vi "SISE-Monitor110-Demo.vi"() -> ()   [LabVIEW 2024]
uses:
  Labview-Projects2019/IonFluxProgramms2019/IonFluxMonitor/SubVIs-SISE-Monitor/Control-IonFlux.ctl
  <vilib>/DAQmx/create/channels.llb/DAQmx Create Channel (AI-Voltage-Basic).vi
  <vilib>/Instr/_visa.llb/VISA Configure Serial Port (Instr).vi
  <vilib>/Analysis/NI_AALPro.lvlib
  <vilib>/DAQmx/read.llb/DAQmx Read (Analog 2D DBL NChan NSamp).vi
panel:
  out "Lesepuffer":string
  out "Registerkarte":enum32{"Start", "Record", "Stop"}(tab)
  out "Output V ch 2":bool
  in  "V channel 2":bool
  out "Output V ch 1":bool
  in  "V channel 1":bool
  out "SISE channel 1":bool
  out "Output SISE ch 2":bool
  in  "SISE channel 2":bool
  out "slow":bool
  in  "Scan angle (degrees)":dbl(slide) scale=0.0..90.0
  out "?":dbl
  in  "VISA res. name":refnum<visa-resource-name> caption="VISA-Ressourcenname"
  in  "Start measurement":bool
  out "Data File":bool
  out "Ind. Channel In":bool
  in  "Data file":path
  out "Ind. Channel Out":bool
  out "?":dbl
  out "Record period (round at 5s)":dbl
  in  "Scan distance (µm)":dbl(slide)=50.0 scale=0.0..100.0
  in  "Record period (single track, s)":dbl(slide)=10.112359550561797 scale=0.0..60.0 scale format="%#_2f"
  in  "Manipulator Speed":bool
  out "fast":bool
  in  "Channels In":tag
  in  "Position of manipulator":bool
  out "left":bool
  out "right":bool
  in  "TC 3":T1(tab)
  in  "Range limit\nS1.1 (mV)":dbl(slide)=200.0 min=0.0 max=600.0 scale=0.2..600.0
  in  "Base line\nS1.1 (mV)":dbl(slide) scale=-300.0..300.0
  in  "Range limit\nS1.2 mV":dbl(slide)=30.0 scale=0.1..30.0
  in  "Base line \nS1.2 (mV)":dbl(slide) scale=-15.0..15.0
  out "dV-SISE channel 1":cluster{dbl[], dbl[]}[](graph)
  out "V-SISE channel 1":cluster{dbl[], dbl[]}[](graph)
  out "V-SISE channel 2":cluster{dbl[], dbl[]}[](graph)
  out "dV-SISE channel 2":cluster{dbl[], dbl[]}[](graph)
  in  "Range limit\nS2.1 (mV)":dbl(slide)=200.0 min=0.0 max=600.0 scale=0.2..600.0
  in  "Base line\nS2.1 (mV)":dbl(slide) scale=-300.0..300.0
  in  "Base line \nS2.2 (mV)":dbl(slide) scale=-15.0..15.0
  in  "Range limit\nS2.2 (mV)":dbl(slide)=30.0 scale=0.1..30.0
  out "Voltage channel 1":cluster{dbl[], dbl[]}[](graph)
  in  "Base line\nV1 (V)":dbl(slide) scale=-300.0..300.0
  in  "Range limit\nV1 (V)":dbl(slide)=200.0 min=0.0 max=600.0 scale=0.2..600.0
  in  "Base line\nV2 (V)":dbl(slide) scale=-300.0..300.0
  in  "Range limit\nV2 (V)":dbl(slide)=200.0 min=0.0 max=600.0 scale=0.2..600.0
  out "Voltage channel 2":cluster{dbl[], dbl[]}[](graph)
  out "V channel #2":bool
  out "V channel #1":bool
  out "SISE channel #2":bool
  out "SISE channel #1":bool
  in  "?":T2(tab)
  in  "V SISE\nch #1":dbl(slide)=4.96774193548387 scale=-10.0..10.0
  out "Vprobe SISE 1":cluster{dbl[], dbl[]}[](graph)
  in  "V SISE\nch #2":dbl(slide)=4.96774193548387 scale=-10.0..10.0
  out "Vprobe SISE 2":cluster{dbl[], dbl[]}[](graph)
  in  "Vch #1":dbl(slide)=5.096774193548386 scale=-10.0..10.0
  out "Vprobe V 1":cluster{dbl[], dbl[]}[](graph)
  in  "Vch\n#2":dbl(slide)=5.096774193548386 scale=-10.0..10.0
  out "Vprobe V 2":cluster{dbl[], dbl[]}[](graph)
  in  "Enable change position 0":bool
  out "Raw data file":path
  in  "Stop measurent":bool
  out "Position probe":cluster{dbl[], dbl[]}[](graph)
  in  "Add Mark":bool
  in  "Event Mark":string
  out "Stop recording":bool
  out "String":string
  out "E-mark on":T3
  out "?":string
  in  "Bildlaufleiste":i32(c297)
  in  "Start fit (% of rec. period)":dbl(slide)=50.0 scale=0.0..100.0
  in  "?":enum32{"dV SISE 1", "dV SISE 2"}(tab)
  out "deltaV SISE 1":cluster{dbl[], "Best Linear Fit":dbl[]}[](graph)
  out "deltaV SISE 2":cluster{dbl[], "Best Linear Fit":dbl[]}[](graph)
  in  "Zoom from start":dbl(slide) scale=0.0..100.0
  in  "Zoom from end":dbl(slide)=100.0 scale=0.0..100.0
  in  "Stop programm":bool
  in  "New measurement":bool
  out "Stop recording 2":bool
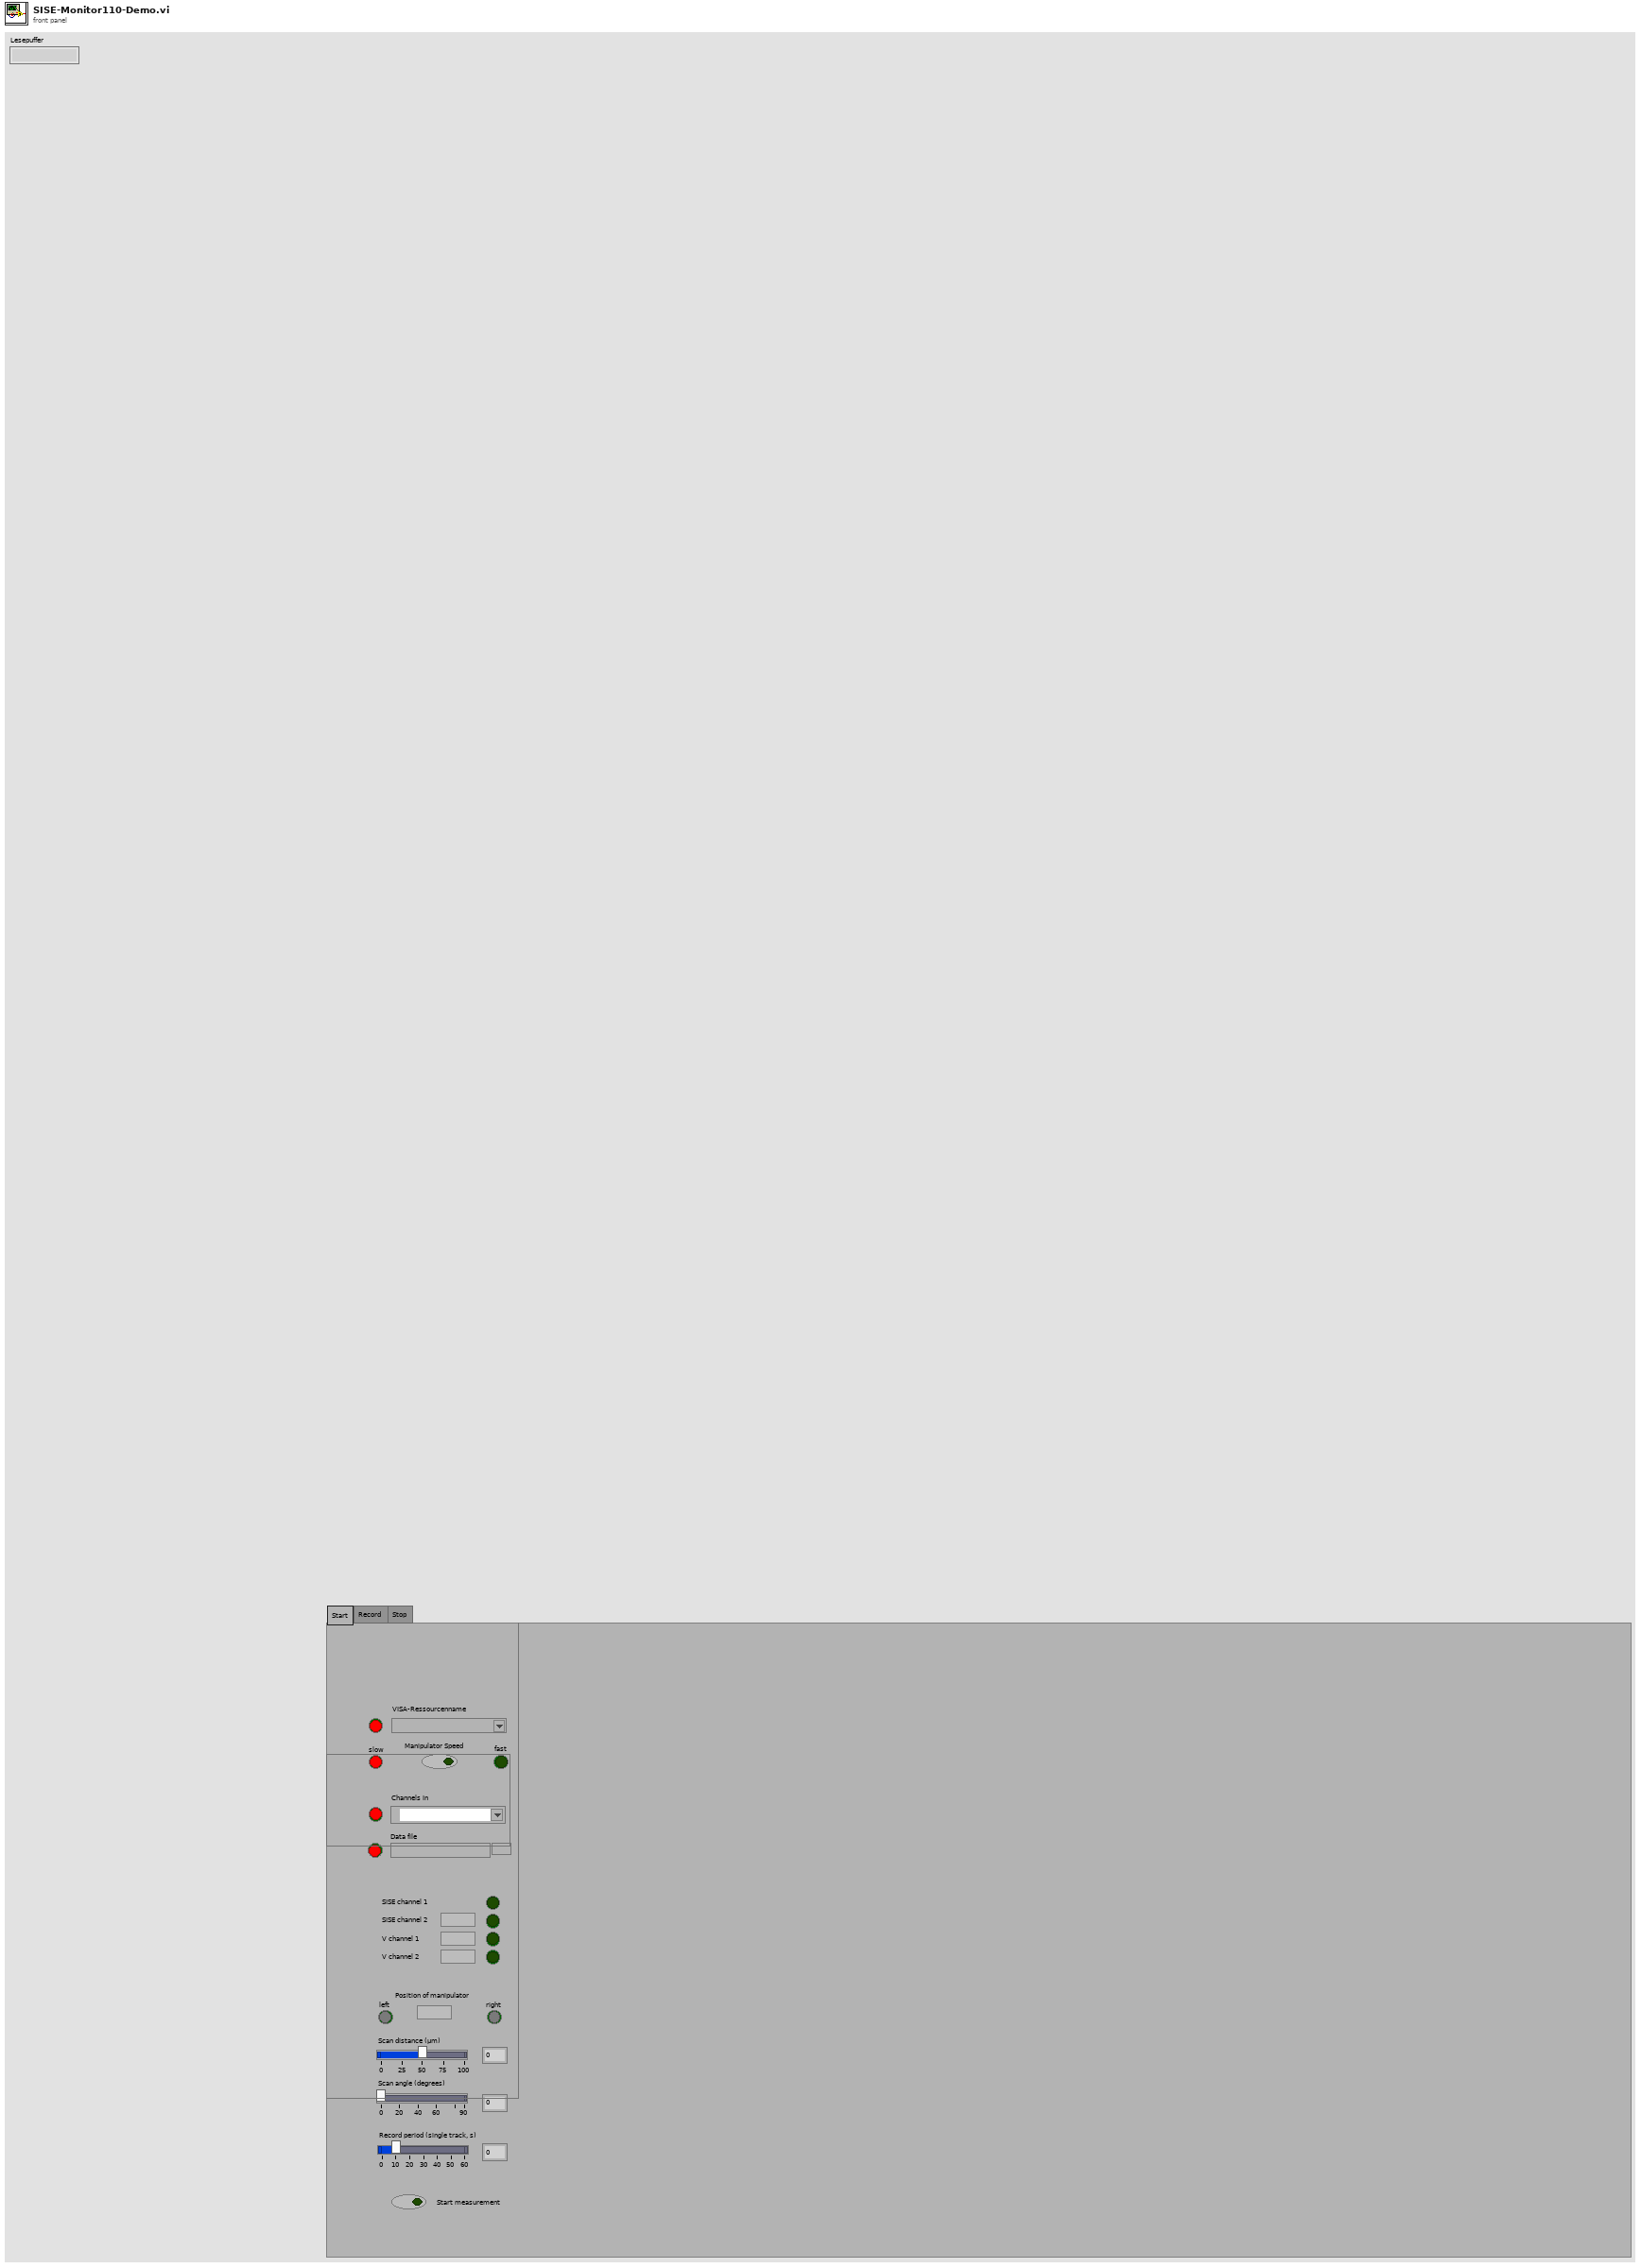
[diagram p1: front panel]
types:
  T1 = enum32{"SISE channel #1", "SISE channel #2", "V channel #1", "V channel #2"}
  T2 = enum32{"SISE chan #1", "SISE chan #2", "V chan #1", "V chan #2"}
  T3 = typedef "Control-IonFlux.ctl" = bool
  T4 = cluster{"refnum out":refnum<file>, "status":bool, "code":i32, "source":string}
  T5 = cluster{"task out":refnum<k21>, "status":bool, "code":i32, "source":string}
  T6 = enum16{"open", "replace", "create", "open or create", "replace or create", "replace or create with confirmation"}
  T7 = cluster{"refnum":refnum<file>, "status":bool, "code":i32, "source":string}
  T8 = cluster{dbl[], dbl[], "Best Linear Fit":dbl[], dbl[], dbl[]}
  T9 = cluster{"Array (Ausgang)":dbl[], "Array (Ausgang)":dbl[]}
  T10 = cluster{"Array (Ausgang)":dbl[], "Array (Ausgang)":dbl[]}[]
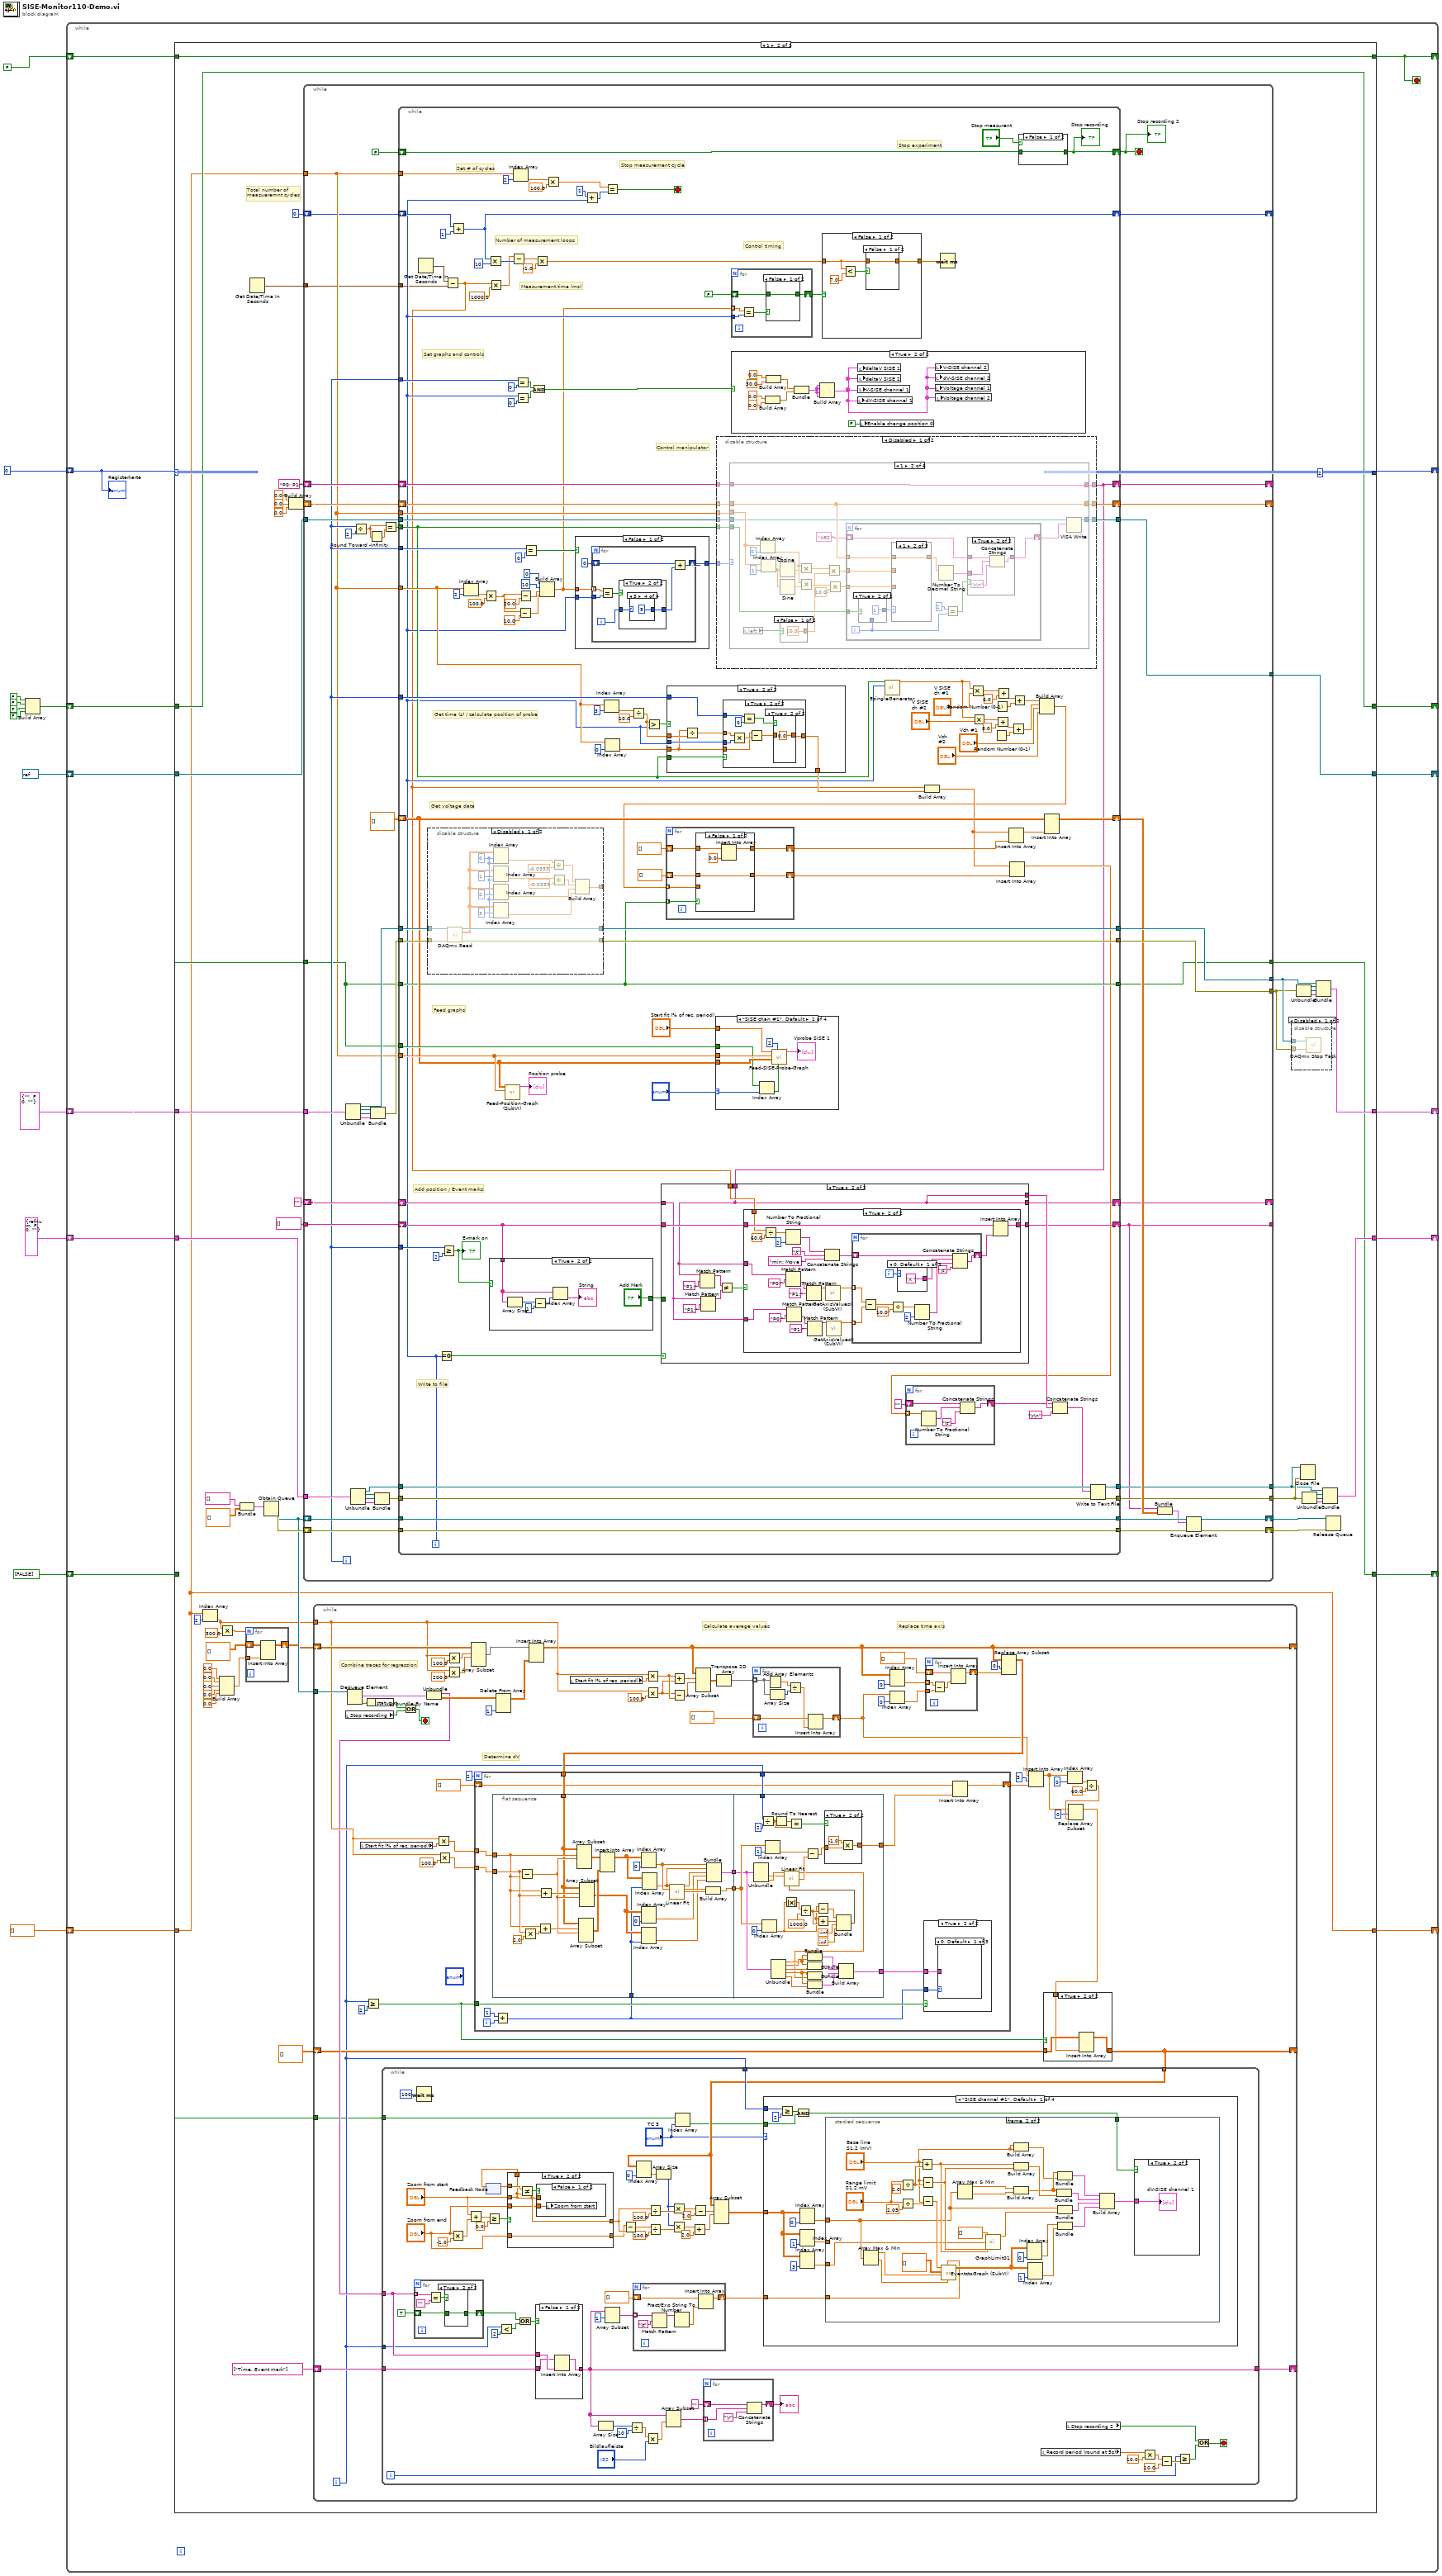
[diagram p0: block diagram]
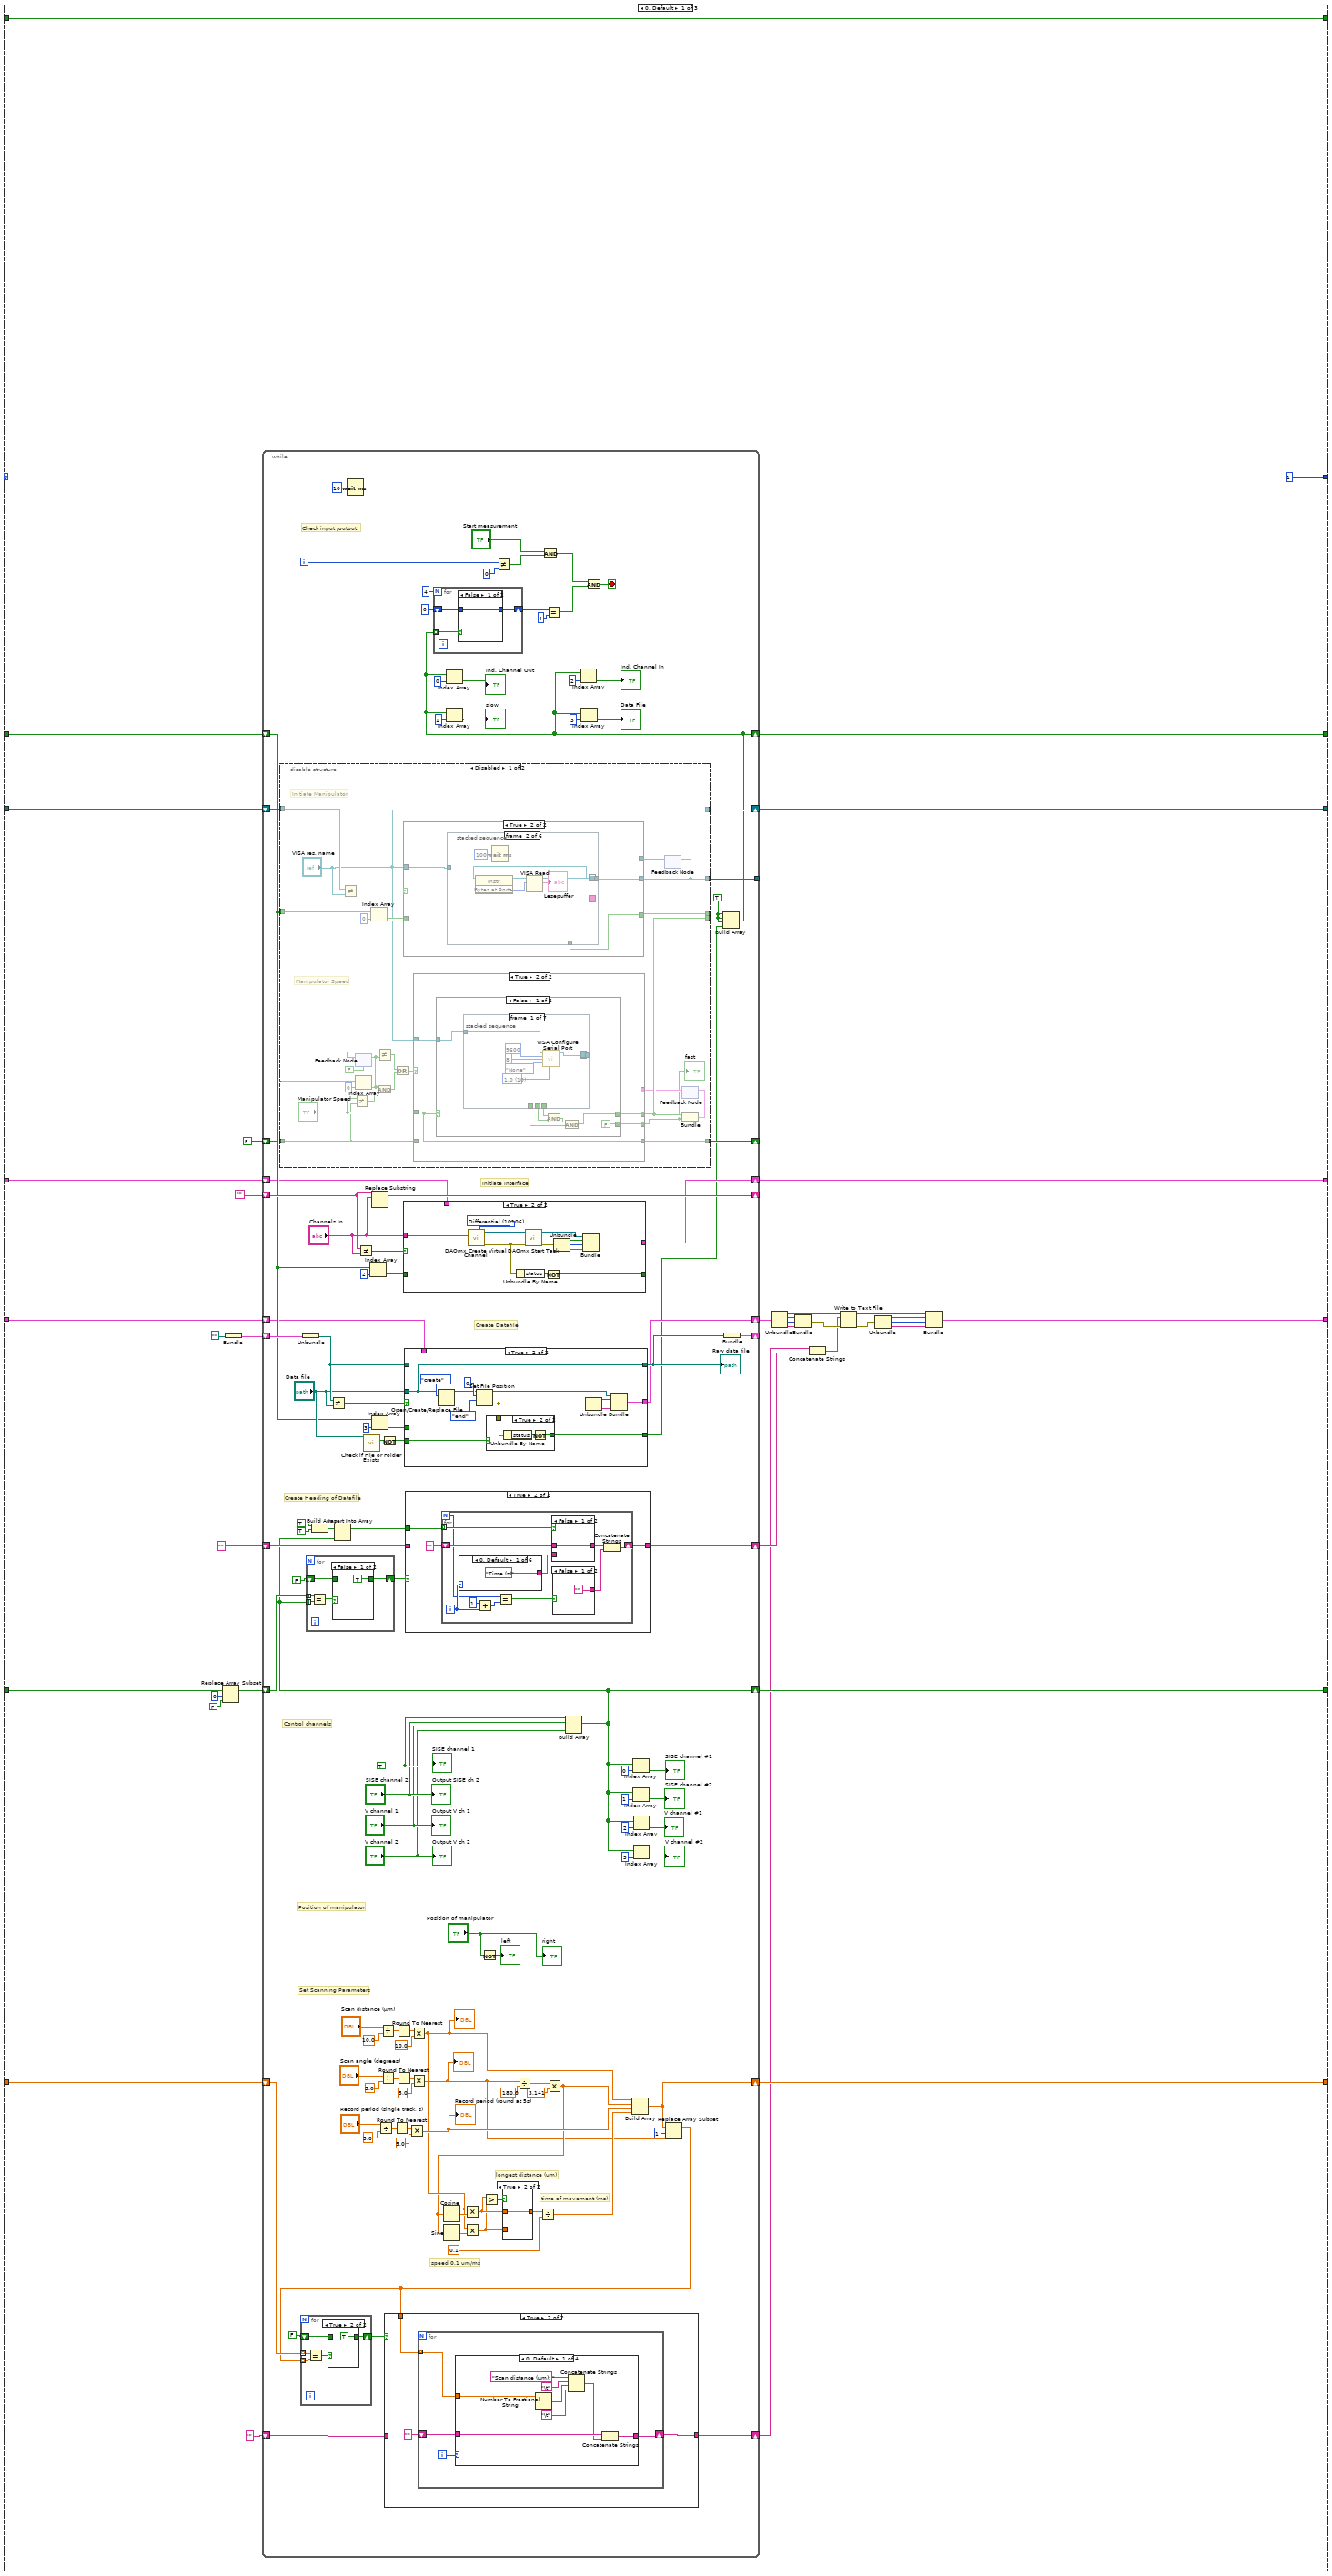
[diagram p2: hidden frame]
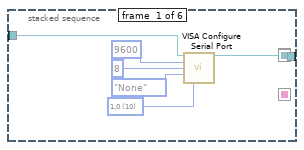
[diagram p4: hidden frame]
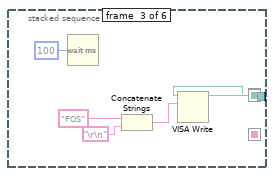
[diagram p5: hidden frame]
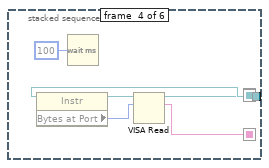
[diagram p6: hidden frame]
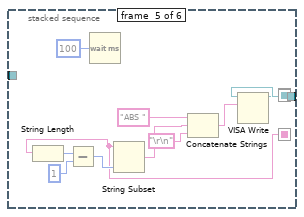
[diagram p7: hidden frame]
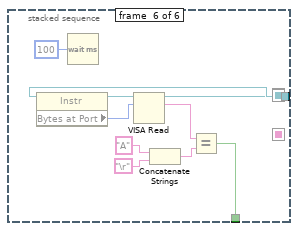
[diagram p8: hidden frame]
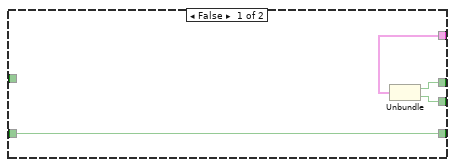
[diagram p9: hidden frame]
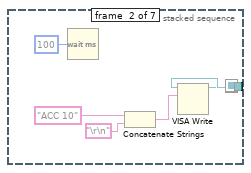
[diagram p10: hidden frame]
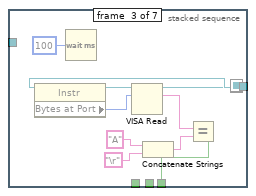
[diagram p11: hidden frame]
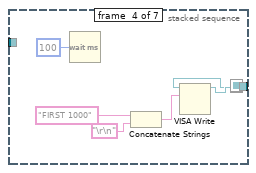
[diagram p12: hidden frame]
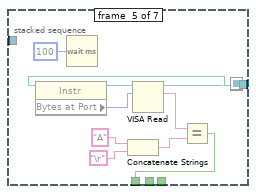
[diagram p13: hidden frame]
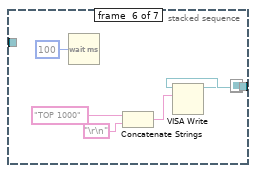
[diagram p14: hidden frame]
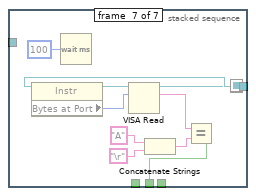
[diagram p15: hidden frame]
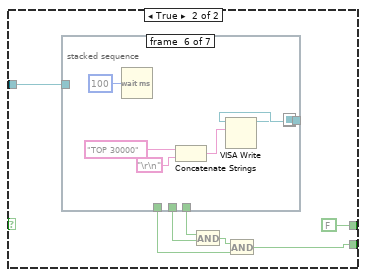
[diagram p16: hidden frame]
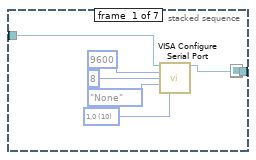
[diagram p17: hidden frame]
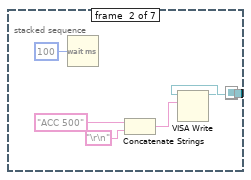
[diagram p18: hidden frame]
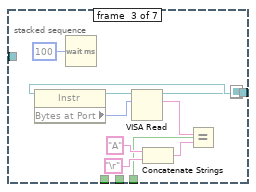
[diagram p19: hidden frame]
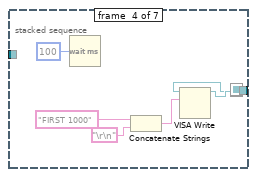
[diagram p20: hidden frame]
diagram:
  n1 = Build Array(FALSE, FALSE, FALSE, FALSE) -> (w1:bool[])
  n2 = while {
    shift-right: [w28] -> _
    shift-left: 0 -> [w27]
    shift-right: [w25] -> _
    shift-left: refnum<visa-resource-name> refnum ("VISA res. name") -> [w26]
    shift-right: [w23] -> _
    shift-left: T5 {"task out"="", "status"=FALSE, "code"=0, "source"=""} -> [w24]
    shift-right: [w19] -> _
    shift-left: T4 {"refnum out"=refnum, "status"=FALSE, "code"=0, "source"=""} -> [w20]
    shift-right: [w22] -> _
    shift-left: dbl[] [] -> [w21]
    shift-right: [w18] -> _
    shift-left: bool[] [FALSE] -> [w17]
    shift-right: [w15] -> _
    shift-left: FALSE -> [w16]
    shift-right: [w13] -> _
    shift-left: w1 -> [w14]
    stop <- w15 stop-if-true
    n3 = case shown="1" w27 {
      tunnel: [1 2 0] -> w28
      tunnel: w26 -> [w60 w561 w1653]
      tunnel: [w59 w560 w1653] -> w25
      tunnel: w24 -> [w58 w559 w1652]
      tunnel: [w57 w555 w1652] -> w23
      tunnel: [w40 w535 w1650] -> w19
      tunnel: w20 -> [w56 w539 w1650]
      tunnel: [w55 w518 w1651] -> w22
      tunnel: w21 -> [w54 w518 w1651]
      tunnel: w17 -> [w31 w525 w1649]
      tunnel: [w53 w532 w1649] -> w18
      tunnel: w16 -> [w39 w524 w1648]
      tunnel: [w39 w524 w1647] -> w15
      tunnel: w14 -> [w33 w523 w1646]
      tunnel: [w38 w523 w1646] -> w13
      frame 0, Default {
        n4 = Replace Array Subset(array=w31, new element=FALSE ("Neues Element/Teil-Array"), index=0 ("Index")) -> (w32:bool[])
        n5 = Bundle(path "") -> (w61:cluster{path})  [unwired: 1 in]
        n6 = while {
          shift-right: [w117] -> w59
          shift-left: w60 -> [w165]
          shift-right: [w90] -> w38
          shift-left: w33 -> [w123]
          tunnel: [w124] -> _
          shift-right: [w160] -> _
          shift-left: "" -> [w159]
          shift-right: [w151] -> _
          shift-left: w61 -> [w153]
          shift-right: [w118] -> _
          shift-left: FALSE -> [w122]
          shift-right: [w115] -> w57
          shift-left: w58 -> [w116]
          shift-right: [w113] -> w51
          shift-left: w56 -> [w112]
          shift-right: [w73] -> w55
          shift-left: w54 -> [w77]
          shift-right: [w82] -> w53
          shift-left: w32 -> [w85]
          shift-right: [w87] -> w36
          shift-left: "" -> [w86]
          shift-right: [w79] -> w35
          shift-left: "" -> [w75]
          i -> [w80]
          stop <- w83 stop-if-true
          w68 = TRUE
          w108 = TRUE
          # "Position of manipulator"
          # "Set Scanning Parameters"
          # "Control channels"
          # "Create Heading of Datafile"
          # "Create Datafile"
          # "Initiate Interface"
          # "Check input /output"
          # "speed 0.1 um/ms"
          # "longest distance (um)"
          # "time of movement (ms)"
          n7 = disable-structure shown="Disabled" {
            disable-tunnel: w165 -> [w200 _]
            disable-tunnel: [w196 _] -> w124
            disable-tunnel: w123 -> [w194 _]
            disable-tunnel: w122 -> [w191 _]
            disable-tunnel: [w184 _] -> _
            disable-tunnel: [w183 _] -> _
            disable-tunnel: [w180 _] -> w118
            disable-tunnel: ["VISA res. name" _] -> w117
            frame Disabled {
              # "Manipulator Speed"
              # "Initiate Manipulator"
              n8 = Not Equal?(x=w200, y="VISA res. name") -> (x != y?=w177:bool)
              n9 = Not Equal?(x="Manipulator Speed", y=w191) -> (x != y?=w193:bool)
              n10 = feedback #1(FALSE) -> (w188:bool)
              n11 = Index Array(array=w194, index=0 ("Index")) -> (element=w189:bool)
              n12 = feedback-in #1(w189) -> ()
              n13 = Index Array(array=w194, index=0 ("Index")) -> (element=w198:bool)
              n14 = Not Equal?(x=w188, y=w189) -> (x != y?=w187:bool)
              n15 = And(x=w189, y=w193) -> (x .and. y?=w185:bool)
              n16 = Or(x=w187, y=w185) -> (x .or. y?=w186:bool)
              n17 = feedback #2() -> (w197:refnum<visa-resource-name>)  [unwired: 1 in]
              n18 = case shown="True" w177 {
                tunnel: w198 -> [w202 _]
                tunnel: [w202 w205] -> w184
                tunnel: "VISA res. name" -> [_ w204]
                tunnel: [w201 w203] -> w196
                tunnel: w197 -> [w201 _]
                frame False {
                }
                frame True {
                  n19 = stacked-sequence {
                    seq-local: [w206 _ _ _ _ _] -> [_ w213 _ _ _ _]
                    seq-local: [_ w214 _ _ _ _] -> [_ _ w218 _ _ _]
                    seq-local: [_ _ w219 _ _ _] -> [_ _ _ w226 _ _]
                    seq-local: [_ _ _ w225 _ _] -> [_ _ _ _ w237 _]
                    seq-local: [_ _ _ w224 _ _] -> [_ _ _ _ w231 _]
                    seq-local: [_ _ _ _ w236 _] -> [_ _ _ _ _ w247]
                    tunnel: w204 -> [w211 _ _ _ _ _]
                    tunnel: [_ _ _ _ _ w246] -> w203
                    tunnel: [_ _ _ _ _ w241] -> w205
                    frame #0 {
                      w207 = u16 10 items=["1,0"=10, "1,5"=15, "2,0"=20] ("stop bits (10: 1 bit)")
                      n20 = call-poly "VISA Configure Serial Port"("VISA resource name"=w211, "baud rate (9600)"=u32 9600, "data bits (8)"=u16 8, "parity (0:none)"=enum16{"None", "Odd", "Even", "Mark", "Space"}."None", "stop bits (10: 1 bit)"=w207) -> ("VISA resource name out"=w206:refnum<visa-resource-name>)  [unwired: 9 in, 1 out]
                    }
                    frame #1 {
                      n21 = property class="Instr"(reference=w213) -> (reference out=w216:refnum<visa-resource-name>, "Bytes at Port"=w215:u32)  [unwired: 1 in, 1 out]
                      n22 = Wait (ms)(milliseconds to wait=u32 100) -> ()  [unwired: 1 out]
                      n23 = VISA Read(VISA resource name=w216, byte count=w215) -> (VISA resource name out=w214:refnum<visa-resource-name>, read buffer=→"Lesepuffer":string)  [unwired: 1 in, 2 out]
                    }
                    frame #2 {
                      n24 = Wait (ms)(milliseconds to wait=u32 100) -> ()  [unwired: 1 out]
                      n25 = Concatenate Strings("POS", "\r\n") -> (w220:string)
                      n26 = VISA Write(VISA resource name=w218, write buffer=w220) -> (VISA resource name out=w219:refnum<visa-resource-name>)  [unwired: 1 in, 2 out]
                    }
                    frame #3 {
                      n27 = property class="Instr"(reference=w226) -> (reference out=w227:refnum<visa-resource-name>, "Bytes at Port"=w228:u32)  [unwired: 1 in, 1 out]
                      n28 = Wait (ms)(milliseconds to wait=u32 100) -> ()  [unwired: 1 out]
                      n29 = VISA Read(VISA resource name=w227, byte count=w228) -> (VISA resource name out=w225:refnum<visa-resource-name>, read buffer=w224:string)  [unwired: 1 in, 2 out]
                    }
                    frame #4 {
                      n30 = String Length(string=w231) -> (length=w234:i32)
                      n31 = Subtract(x=w234, y=1) -> (x-y=w232:i32)
                      n32 = Wait (ms)(milliseconds to wait=u32 100) -> ()  [unwired: 1 out]
                      n33 = String Subset(string=w231, length (rest)=w232) -> (substring=w230:string)  [unwired: 1 in]
                      n34 = Concatenate Strings("ABS ", w230, "\r\n") -> (w238:string)
                      n35 = VISA Write(VISA resource name=w237, write buffer=w238) -> (VISA resource name out=w236:refnum<visa-resource-name>)  [unwired: 1 in, 2 out]
                    }
                    frame #5 {
                      n36 = property class="Instr"(reference=w247) -> (reference out=w248:refnum<visa-resource-name>, "Bytes at Port"=w249:u32)  [unwired: 1 in, 1 out]
                      n37 = Wait (ms)(milliseconds to wait=u32 100) -> ()  [unwired: 1 out]
                      n38 = VISA Read(VISA resource name=w248, byte count=w249) -> (VISA resource name out=w246:refnum<visa-resource-name>, read buffer=w242:string)  [unwired: 1 in, 2 out]
                      n39 = Concatenate Strings("A", "\r") -> (w245:string)
                      n40 = Equal?(x=w242, y=w245) -> (x = y?=w241:bool)
                    }
                  }
                }
              }
              n41 = feedback-in #2(w196) -> ()
              n42 = feedback #3() -> (w181:cluster{bool, bool})  [unwired: 1 in]
              n43 = case shown="True" w186 {
                tunnel: "VISA res. name" -> [_ w258]
                tunnel: [w254 w257] -> w180
                tunnel: "Manipulator Speed" -> [_ w257]
                tunnel: w191 -> [w254 _]
                tunnel: [w251 w256] -> w183
                tunnel: [w252 w255] -> w178
                tunnel: w181 -> [w253 _]
                frame False {
                  n44 = Unbundle(w253) -> (w251:bool, w252:bool)
                }
                frame True {
                  n45 = case shown="False" w257 {
                    tunnel: w258 -> [w265 w326]
                    tunnel: [FALSE w320] -> w255
                    tunnel: [w259 FALSE] -> w256
                    frame False {
                      n46 = stacked-sequence {
                        seq-local: [w266 _ _ _ _ _ _] -> [_ w276 _ _ _ _ _]
                        seq-local: [_ w272 _ _ _ _ _] -> [_ _ w285 _ _ _ _]
                        seq-local: [_ _ w279 _ _ _ _] -> [_ _ _ w288 _ _ _]
                        seq-local: [_ _ _ w289 _ _ _] -> [_ _ _ _ w300 _ _]
                        seq-local: [_ _ _ _ w299 _ _] -> [_ _ _ _ _ w305 _]
                        seq-local: [_ _ _ _ _ w304 _] -> [_ _ _ _ _ _ w316]
                        tunnel: w265 -> [w271 _ _ _ _ _ _]
                        tunnel: [_ _ w278 _ _ _ _] -> w263
                        tunnel: [_ _ _ _ w294 _ _] -> w261
                        tunnel: [_ _ _ _ _ _ w315] -> _
                        tunnel: [_ _ _ _ _ _ w310] -> w262
                        frame #0 {
                          w267 = u16 10 items=["1,0"=10, "1,5"=15, "2,0"=20] ("stop bits (10: 1 bit)")
                          n47 = call-poly "VISA Configure Serial Port"("VISA resource name"=w271, "baud rate (9600)"=u32 9600, "data bits (8)"=u16 8, "parity (0:none)"=enum16{"None", "Odd", "Even", "Mark", "Space"}."None", "stop bits (10: 1 bit)"=w267) -> ("VISA resource name out"=w266:refnum<visa-resource-name>)  [unwired: 9 in, 1 out]
                        }
                        frame #1 {
                          n48 = Wait (ms)(milliseconds to wait=u32 100) -> ()  [unwired: 1 out]
                          n49 = Concatenate Strings("ACC 10", "\r\n") -> (w273:string)
                          n50 = VISA Write(VISA resource name=w276, write buffer=w273) -> (VISA resource name out=w272:refnum<visa-resource-name>)  [unwired: 1 in, 2 out]
                        }
                        frame #2 {
                          n51 = property class="Instr"(reference=w285) -> (reference out=w286:refnum<visa-resource-name>, "Bytes at Port"=w284:u32)  [unwired: 1 in, 1 out]
                          n52 = Wait (ms)(milliseconds to wait=u32 100) -> ()  [unwired: 1 out]
                          n53 = VISA Read(VISA resource name=w286, byte count=w284) -> (VISA resource name out=w279:refnum<visa-resource-name>, read buffer=w283:string)  [unwired: 1 in, 2 out]
                          n54 = Concatenate Strings("A", "\r") -> (w280:string)
                          n55 = Equal?(x=w283, y=w280) -> (x = y?=w278:bool)
                        }
                        frame #3 {
                          n56 = Wait (ms)(milliseconds to wait=u32 100) -> ()  [unwired: 1 out]
                          n57 = Concatenate Strings("FIRST 1000", "\r\n") -> (w290:string)
                          n58 = VISA Write(VISA resource name=w288, write buffer=w290) -> (VISA resource name out=w289:refnum<visa-resource-name>)  [unwired: 1 in, 2 out]
                        }
                        frame #4 {
                          n59 = property class="Instr"(reference=w300) -> (reference out=w301:refnum<visa-resource-name>, "Bytes at Port"=w302:u32)  [unwired: 1 in, 1 out]
                          n60 = Wait (ms)(milliseconds to wait=u32 100) -> ()  [unwired: 1 out]
                          n61 = Concatenate Strings("A", "\r") -> (w295:string)
                          n62 = VISA Read(VISA resource name=w301, byte count=w302) -> (VISA resource name out=w299:refnum<visa-resource-name>, read buffer=w298:string)  [unwired: 1 in, 2 out]
                          n63 = Equal?(x=w298, y=w295) -> (x = y?=w294:bool)
                        }
                        frame #5 {
                          n64 = Wait (ms)(milliseconds to wait=u32 100) -> ()  [unwired: 1 out]
                          n65 = Concatenate Strings("TOP 1000", "\r\n") -> (w306:string)
                          n66 = VISA Write(VISA resource name=w305, write buffer=w306) -> (VISA resource name out=w304:refnum<visa-resource-name>)  [unwired: 1 in, 2 out]
                        }
                        frame #6 {
                          n67 = property class="Instr"(reference=w316) -> (reference out=w317:refnum<visa-resource-name>, "Bytes at Port"=w318:u32)  [unwired: 1 in, 1 out]
                          n68 = Wait (ms)(milliseconds to wait=u32 100) -> ()  [unwired: 1 out]
                          n69 = VISA Read(VISA resource name=w317, byte count=w318) -> (VISA resource name out=w315:refnum<visa-resource-name>, read buffer=w311:string)  [unwired: 1 in, 2 out]
                          n70 = Concatenate Strings("A", "\r") -> (w314:string)
                          n71 = Equal?(x=w311, y=w314) -> (x = y?=w310:bool)
                        }
                      }
                      n72 = And(x=w263, y=w262) -> (x .and. y?=w264:bool)
                      n73 = And(x=w264, y=w261) -> (x .and. y?=w259:bool)
                    }
                    frame True {
                      n74 = stacked-sequence {
                        seq-local: [w327 _ _ _ _ _ _] -> [_ w337 _ _ _ _ _]
                        seq-local: [_ w333 _ _ _ _ _] -> [_ _ w346 _ _ _ _]
                        seq-local: [_ _ w340 _ _ _ _] -> [_ _ _ w349 _ _ _]
                        seq-local: [_ _ _ w350 _ _ _] -> [_ _ _ _ w361 _ _]
                        seq-local: [_ _ _ _ w360 _ _] -> [_ _ _ _ _ w366 _]
                        seq-local: [_ _ _ _ _ w365 _] -> [_ _ _ _ _ _ w377]
                        tunnel: w326 -> [w332 _ _ _ _ _ _]
                        tunnel: [_ _ w339 _ _ _ _] -> w324
                        tunnel: [_ _ _ _ w355 _ _] -> w322
                        tunnel: [_ _ _ _ _ _ w376] -> _
                        tunnel: [_ _ _ _ _ _ w371] -> w323
                        frame #0 {
                          w328 = u16 10 items=["1,0"=10, "1,5"=15, "2,0"=20] ("stop bits (10: 1 bit)")
                          n75 = call-poly "VISA Configure Serial Port"("VISA resource name"=w332, "baud rate (9600)"=u32 9600, "data bits (8)"=u16 8, "parity (0:none)"=enum16{"None", "Odd", "Even", "Mark", "Space"}."None", "stop bits (10: 1 bit)"=w328) -> ("VISA resource name out"=w327:refnum<visa-resource-name>)  [unwired: 9 in, 1 out]
                        }
                        frame #1 {
                          n76 = Wait (ms)(milliseconds to wait=u32 100) -> ()  [unwired: 1 out]
                          n77 = Concatenate Strings("ACC 500", "\r\n") -> (w334:string)
                          n78 = VISA Write(VISA resource name=w337, write buffer=w334) -> (VISA resource name out=w333:refnum<visa-resource-name>)  [unwired: 1 in, 2 out]
                        }
                        frame #2 {
                          n79 = property class="Instr"(reference=w346) -> (reference out=w347:refnum<visa-resource-name>, "Bytes at Port"=w345:u32)  [unwired: 1 in, 1 out]
                          n80 = Wait (ms)(milliseconds to wait=u32 100) -> ()  [unwired: 1 out]
                          n81 = VISA Read(VISA resource name=w347, byte count=w345) -> (VISA resource name out=w340:refnum<visa-resource-name>, read buffer=w344:string)  [unwired: 1 in, 2 out]
                          n82 = Concatenate Strings("A", "\r") -> (w341:string)
                          n83 = Equal?(x=w344, y=w341) -> (x = y?=w339:bool)
                        }
                        frame #3 {
                          n84 = Wait (ms)(milliseconds to wait=u32 100) -> ()  [unwired: 1 out]
                          n85 = Concatenate Strings("FIRST 1000", "\r\n") -> (w351:string)
                          n86 = VISA Write(VISA resource name=w349, write buffer=w351) -> (VISA resource name out=w350:refnum<visa-resource-name>)  [unwired: 1 in, 2 out]
                        }
                        frame #4 {
                          n87 = property class="Instr"(reference=w361) -> (reference out=w362:refnum<visa-resource-name>, "Bytes at Port"=w363:u32)  [unwired: 1 in, 1 out]
                          n88 = Wait (ms)(milliseconds to wait=u32 100) -> ()  [unwired: 1 out]
                          n89 = Concatenate Strings("A", "\r") -> (w356:string)
                          n90 = VISA Read(VISA resource name=w362, byte count=w363) -> (VISA resource name out=w360:refnum<visa-resource-name>, read buffer=w359:string)  [unwired: 1 in, 2 out]
                          n91 = Equal?(x=w359, y=w356) -> (x = y?=w355:bool)
                        }
                        frame #5 {
                          n92 = Wait (ms)(milliseconds to wait=u32 100) -> ()  [unwired: 1 out]
                          n93 = Concatenate Strings("TOP 30000", "\r\n") -> (w367:string)
                          n94 = VISA Write(VISA resource name=w366, write buffer=w367) -> (VISA resource name out=w365:refnum<visa-resource-name>)  [unwired: 1 in, 2 out]
                        }
                        frame #6 {
                          n95 = property class="Instr"(reference=w377) -> (reference out=w378:refnum<visa-resource-name>, "Bytes at Port"=w379:u32)  [unwired: 1 in, 1 out]
                          n96 = Wait (ms)(milliseconds to wait=u32 100) -> ()  [unwired: 1 out]
                          n97 = VISA Read(VISA resource name=w378, byte count=w379) -> (VISA resource name out=w376:refnum<visa-resource-name>, read buffer=w372:string)  [unwired: 1 in, 2 out]
                          n98 = Concatenate Strings("A", "\r") -> (w375:string)
                          n99 = Equal?(x=w372, y=w375) -> (x = y?=w371:bool)
                        }
                      }
                      n100 = And(x=w324, y=w323) -> (x .and. y?=w325:bool)
                      n101 = And(x=w325, y=w322) -> (x .and. y?=w320:bool)
                    }
                  }
                }
              }
              "fast" <- w178
              n102 = Bundle(w183, w178) -> (w182:cluster{bool, bool})  [unwired: 1 in]
              n103 = feedback-in #3(w182) -> ()
            }
            frame Enabled {
            }
          }
          n104 = Unbundle(w153) -> (w152:path)
          n105 = Build Array(TRUE, TRUE) -> (w93:bool[])
          n106 = Not Equal?(x=w152, y="Data file") -> (x != y?=w92:bool)
          n107 = Wait (ms)(milliseconds to wait=u32 10) -> ()  [unwired: 1 out]
          n108 = Not Equal?(x=w159, y="Channels In") -> (x != y?=w162:bool)
          n109 = call <vilib>:"Check if File or Folder Exists.vi"("path"="Data file") -> ("file or folder exists?"=w157:bool)  [unwired: 8 in, 2 out]
          n110 = Index Array(array=w123, index=2 ("Index")) -> (element=w161:bool)
          n111 = Replace Substring(4:"Channels In", 5:w159) -> (1:w160:string)  [unwired: 2 in, 1 out]
          n112 = Index Array(array=w123, index=3 ("Index")) -> (element=w154:bool)
          n113 = Divide(x="Record period (single track, s)", y=5.0) -> (x/y=w166:dbl)
          n114 = Divide(x="Scan distance (µm)", y=10.0) -> (x/y=w173:dbl)
          n115 = Divide(x="Scan angle (degrees)", y=5.0) -> (x/y=w141:dbl)
          n116 = Not(x=w157) -> (.not. x?=w149:bool)
          n117 = Round To Nearest(number=w166) -> (nearest integer value=w169:dbl)
          n118 = Round To Nearest(number=w173) -> (nearest integer value=w172:dbl)
          n119 = Round To Nearest(number=w141) -> (nearest integer value=w140:dbl)
          n120 = case shown="True" w162 {
            tunnel: w161 -> [w503 _]
            tunnel: [w503 w514] -> _
            tunnel: "Channels In" -> [_ w505]
            tunnel: w116 -> [w502 _]
            tunnel: [w502 w508] -> w115
            frame False {
            }
            frame True {
              w504 = 10106 items=["Default"=-1, "RSE"=10083, "NRSE"=10078, "Differential"=10106, "Pseudodifferential"=12529] ("input terminal configuration")
              n121 = call-poly <vilib>:"DAQmx Create Virtual Channel.vi"("input terminal configuration"=w504, "physical channels"=w505) -> ("task out"=w507:refnum<k21>, "error out"=w506:errorcluster)  [unwired: 12 in]
              n122 = Unbundle By Name(w506) -> ("status"=w515:bool)
              n123 = call <vilib>:"DAQmx Start Task.vi"("task/channels in"=w507, "error in"=w506) -> ("task out"=w509:refnum<k21>, "error out"=w513:errorcluster)  [unwired: 12 in]
              n124 = Not(x=w515) -> (.not. x?=w514:bool)
              n125 = Unbundle(w513) -> ("status"=w510:bool, "code"=w511:i32, "source"=w512:string)
              n126 = Bundle("task out"=w509, "status"=w510, "code"=w511, "source"=w512) -> (w508:T5)  [unwired: 1 in]
            }
          }
          n127 = case shown="True" w92 {
            tunnel: "Data file" -> [_ w491]
            tunnel: [w483 w492] -> w69
            tunnel: w154 -> [w483 _]
            tunnel: w152 -> [w482 _]
            tunnel: [w482 w491] -> w114
            tunnel: w149 -> [_ w490]
            tunnel: [w481 w486] -> w113
            tunnel: w112 -> [w481 _]
            frame False {
            }
            frame True {
              n128 = Open/Create/Replace File(file path (use dialog)=w491, operation (0:open)=T6."create") -> (refnum out=w495:refnum<file>, error out=w494:errorcluster)  [unwired: 4 in, 1 out]
              n129 = Set File Position(offset (in bytes) (0)=i64 0, refnum=w495, from (0:start)=enum16{"start", "end", "current"}."end", error in=w494) -> (refnum out=w484:refnum<file>, error out=w485:errorcluster)
              n130 = case shown="True" w490 {
                tunnel: [FALSE w500] -> w492
                tunnel: w485 -> [_ w499]
                frame False {
                }
                frame True {
                  n131 = Unbundle By Name(w499) -> ("status"=w501:bool)
                  n132 = Not(x=w501) -> (.not. x?=w500:bool)
                }
              }
              n133 = Unbundle(w485) -> ("status"=w489:bool, "code"=w488:i32, "source"=w487:string)
              n134 = Bundle("refnum"=w484, "status"=w489, "code"=w488, "source"=w487) -> (w486:T7)  [unwired: 1 in]
            }
          }
          "Raw data file" <- w114
          n135 = Multiply(x=w169, y=5.0) -> (x*y=w136:dbl)
          "Record period (round at 5s)" <- w136
          n136 = Multiply(x=w172, y=10.0) -> (x*y=w130:dbl)
          "?" <- w130
          n137 = Multiply(x=w140, y=5.0) -> (x*y=w71:dbl)
          "?" <- w71
          n138 = Not(x="Position of manipulator") -> (.not. x?=→"left":bool)
          n139 = Not Equal?(x=w80, y=0) -> (x != y?=w146:bool)
          n140 = Divide(x=w71, y=180.0) -> (x/y=w109:dbl)
          n141 = And(x="Start measurement", y=w146) -> (x .and. y?=w89:bool)
          n142 = Multiply(x=w109, y=3.141) -> (x*y=w74:dbl)
          n143 = Cosine(x=w74) -> (cos(x)=w135:dbl)
          n144 = Sine(x=w74) -> (sin(x)=w134:dbl)
          n145 = Multiply(x=w130, y=w135) -> (x*y=w133:dbl)
          n146 = Multiply(x=w130, y=w134) -> (x*y=w132:dbl)
          n147 = Greater?(x=w133, y=w132) -> (0:w131:bool)
          n148 = case shown="True" w131 {
            tunnel: w133 -> [_ w473]
            tunnel: w132 -> [w472 _]
            tunnel: [w472 w473] -> w129
            frame False {
            }
            frame True {
            }
          }
          n149 = Divide(x=w129, y=0.1) -> (x/y=w127:dbl)
          n150 = Build Array(w108, "SISE channel 2", "V channel 1", "V channel 2") -> (w82:bool[])
          n151 = for {
            tunnel: w85 -> [w432] mode=indexing
            tunnel: w82 -> [w431] mode=indexing
            shift-right: [w428] -> w81
            shift-left: FALSE -> [w429]
            n152 = Equal?(x=w432, y=w431) -> (x = y?=w430:bool)
            n153 = case shown="False" w430 {
              tunnel: w429 -> [_ w434]
              tunnel: [TRUE w434] -> w428
              frame False {
              }
              frame True {
              }
            }
          }
          n154 = Insert Into Array(array=w93, new element=w82) -> (w88:bool[])  [unwired: 1 in]
          n155 = case shown="True" w81 {
            tunnel: w88 -> [_ w437]
            tunnel: [w435 w436] -> w87
            tunnel: w86 -> [w435 _]
            frame False {
            }
            frame True {
              n156 = for {
                N -> [w441]
                shift-right: [w446] -> w436
                shift-left: "" -> [w449]
                tunnel: w437 -> [w447] mode=indexing
                i -> [w444]
                n157 = case shown="0, Default" w444 {
                  tunnel: ["Time (s)" w459 w462 w465 w468 w471] -> w448
                  frame 0, Default {
                  }
                  frame 1 {
                    n158 = Concatenate Strings("\t", "Position") -> (w459:string)
                  }
                  frame 2 {
                    n159 = Concatenate Strings("\t", "SISE 1 (mV)") -> (w462:string)
                  }
                  frame 3 {
                    n160 = Concatenate Strings("\t", "SISE 2 (mV)") -> (w465:string)
                  }
                  frame 4 {
                    n161 = Concatenate Strings("\t", "Voltage 1 (V)") -> (w468:string)
                  }
                  frame 5 {
                    n162 = Concatenate Strings("\t", "Voltage 2 (V)") -> (w471:string)
                  }
                }
                n163 = Add(x=1, y=w444) -> (x+y=w442:i32)
                n164 = Equal?(x=w441, y=w442) -> (x = y?=w440:bool)
                n165 = case shown="False" w447 {
                  tunnel: w449 -> [w452 w455]
                  tunnel: [w452 w454] -> w445
                  tunnel: w448 -> [_ w453]
                  frame False {
                  }
                  frame True {
                    n166 = Concatenate Strings(w455, w453) -> (w454:string)
                  }
                }
                n167 = case shown="False" w440 {
                  tunnel: ["" "\r\n"] -> w439
                  frame False {
                  }
                  frame True {
                  }
                }
                n168 = Concatenate Strings(w445, w439) -> (w446:string)
              }
            }
          }
          n169 = Build Array(w130, w74, w136, w127) -> (w73:dbl[])
          n170 = Index Array(array=w82, index=0 ("Index")) -> (element=→"SISE channel #1":bool)
          n171 = Index Array(array=w82, index=1 ("Index")) -> (element=→"SISE channel #2":bool)
          n172 = Index Array(array=w82, index=2 ("Index")) -> (element=→"V channel #1":bool)
          n173 = Index Array(array=w82, index=3 ("Index")) -> (element=→"V channel #2":bool)
          n174 = Replace Array Subset(array=w73, new element=w71, index=1 ("Index")) -> (w70:dbl[])
          n175 = for {
            shift-right: [w421] -> w76
            shift-left: FALSE -> [w422]
            tunnel: w77 -> [w425] mode=indexing
            tunnel: w70 -> [w424] mode=indexing
            n176 = Equal?(x=w425, y=w424) -> (x = y?=w423:bool)
            n177 = case shown="True" w423 {
              tunnel: w422 -> [w426 _]
              tunnel: [w426 TRUE] -> w421
              frame False {
              }
              frame True {
              }
            }
          }
          n178 = case shown="True" w76 {
            tunnel: [w381 w384] -> w79
            tunnel: w70 -> [_ w382]
            tunnel: w75 -> [w381 _]
            frame False {
            }
            frame True {
              n179 = for {
                tunnel: w382 -> [w385] mode=indexing
                shift-right: [w386] -> w384
                shift-left: "" -> [w387]
                i -> [w388]
                n180 = case shown="0, Default" w388 {
                  tunnel: [w396 w398 w408 w416] -> w386
                  tunnel: w387 -> [w395 w399 w407 w413]
                  tunnel: w385 -> [w391 w400 w406 w414]
                  frame 0, Default {
                    n181 = Number To Fractional String(number=w391) -> (F-format string=w390:string)  [unwired: 3 in]
                    n182 = Concatenate Strings("Scan distance (µm): ", "\t", w390, "\t") -> (w392:string)
                    n183 = Concatenate Strings(w395, w392) -> (w396:string)
                  }
                  frame 1 {
                    n184 = Number To Fractional String(number=w400) -> (F-format string=w404:string)  [unwired: 3 in]
                    n185 = Concatenate Strings("Scan angle (degrees): ", "\t", w404, "\t") -> (w397:string)
                    n186 = Concatenate Strings(w399, w397) -> (w398:string)
                  }
                  frame 2 {
                    n187 = Number To Fractional String(number=w406) -> (F-format string=w412:string)  [unwired: 3 in]
                    n188 = Concatenate Strings("Record period (single track, s): ", "\t", w412, "\t") -> (w405:string)
                    n189 = Concatenate Strings(w407, w405) -> (w408:string)
                  }
                  frame 3 {
                    n190 = Number To Fractional String(number=w414) -> (F-format string=w420:string)  [unwired: 3 in]
                    n191 = Concatenate Strings("Time of movement (ms): ", "\t", w420, "\r\n") -> (w415:string)
                    n192 = Concatenate Strings(w413, w415) -> (w416:string)
                  }
                }
              }
            }
          }
          n193 = Build Array(w68, w68, w68, w69) -> (w90:bool[])
          n194 = for {
            N: 4 -> [_]
            tunnel: w90 -> [w476] mode=indexing
            shift-right: [w474] -> w91
            shift-left: 0 -> [w475]
            n195 = case shown="False" w476 {
              tunnel: w475 -> [w477 w480]
              tunnel: [w477 w478] -> w474
              frame False {
              }
              frame True {
                n196 = Add(x=w480, y=1) -> (x+y=w478:i32)
              }
            }
          }
          n197 = Index Array(array=w90, index=0 ("Index")) -> (element=→"Ind. Channel Out":bool)
          n198 = Index Array(array=w90, index=1 ("Index")) -> (element=→"slow":bool)
          n199 = Equal?(x=w91, y=4) -> (x = y?=w142:bool)
          n200 = Index Array(array=w90, index=2 ("Index")) -> (element=→"Ind. Channel In":bool)
          n201 = Index Array(array=w90, index=3 ("Index")) -> (element=→"Data File":bool)
          n202 = And(x=w89, y=w142) -> (x .and. y?=w83:bool)
          n203 = Bundle("Data file"=w114) -> (w151:cluster{"Data file ":path})  [unwired: 1 in]
          "Output SISE ch 2" <- "SISE channel 2"
          "SISE channel 1" <- w108
          "Output V ch 1" <- "V channel 1"
          "Output V ch 2" <- "V channel 2"
          "right" <- "Position of manipulator"
        }
        n204 = Unbundle(w51) -> ("refnum out"=w46:refnum<file>, "status"=w50:bool, "code"=w49:i32, "source"=w48:string)
        n205 = Bundle("status"=w50, "code"=w49, "source"=w48) -> (w47:errorcluster)  [unwired: 1 in]
        n206 = Concatenate Strings(w35, w36) -> (w34:string)
        n207 = Write to Text File(file (use dialog)=w46, text=w34, error in=w47) -> (refnum out=w44:refnum<file>, error out=w45:errorcluster)  [unwired: 1 in, 1 out]
        n208 = Unbundle(w45) -> ("status"=w43:bool, "code"=w42:i32, "source"=w41:string)
        n209 = Bundle("refnum out"=w44, "status"=w43, "code"=w42, "source"=w41) -> (w40:T4)  [unwired: 1 in]
      }
      frame 1 {
        # "Total number of \nmeasueremnt cycles"
        n210 = Index Array(array=w518, index=2 ("Index")) -> (element=w545:dbl)
        n211 = Build Array(0.0, 0.0, 0.0, 0.0, 0.0) -> (w526:dbl[])
        n212 = Multiply(x=w545, y=300.0 ("x")) -> (x*y=w549:dbl)
        n213 = Bundle(string[] [], dbl[][] []) -> (w542:cluster{string[], dbl[][]})  [unwired: 1 in]
        n214 = for {
          N: w549 -> [_]
          shift-right: [w572] -> w546
          shift-left: dbl[][] [] -> [w571]
          tunnel: w526 -> [w570]
          n215 = Insert Into Array(array=w571, new element=w570) -> (w572:dbl[][])  [unwired: 2 in]
        }
        n216 = Get Date/Time In Seconds() -> (seconds since 1Jan1904=w516:timestamp)
        n217 = Obtain Queue(element data type=w542) -> (queue out=w551:refnum<queue>, error out=w554:errorcluster)  [unwired: 4 in, 1 out]
        n218 = Build Array(0.0 ("Element"), 0.0 ("Element"), 0.0 ("Element")) -> (w562:dbl[])
        n219 = while {
          tunnel: w561 -> [w1105]
          shift-right: [w1104] -> _
          shift-left: "P0: P1:" -> [w1107]
          shift-right: [w1103] -> _
          shift-left: w562 -> [w1106]
          tunnel: [w1102] -> w560
          tunnel: w559 -> [w1101]
          tunnel: [w1096] -> w522
          tunnel: [w1095] -> w521
          shift-right: [w1090] -> w553
          shift-left: w551 -> [w1088]
          shift-right: [w1089] -> w552
          shift-left: w554 -> [w1093]
          tunnel: w539 -> [w1085]
          tunnel: [w1079] -> w520
          tunnel: [w1078] -> w519
          shift-right: [w1074] -> _
          shift-left: "" -> [w1076]
          tunnel: string[] [] -> [w1077]
          tunnel: [w1075] -> _
          tunnel: w525 -> [w1071]
          tunnel: [w1070] -> w532
          tunnel: w518 -> [w1068]
          shift-right: [w1066] -> _
          shift-left: 0 -> [w1067]
          tunnel: w516 -> [w1065]
          i -> [w1073]
          stop <- w1069 stop-if-true
          n220 = Unbundle(w1101) -> ("task out"=w1072:refnum<k21>, "status"=w1100:bool, "code"=w1099:i32, "source"=w1098:string)
          n221 = Unbundle(w1085) -> ("refnum out"=w1081:refnum<file>, "status"=w1084:bool, "code"=w1082:i32, "source"=w1083:string)
          n222 = Divide(x=w1073, y=2) -> (x/y=w1110:dbl)
          n223 = Round Toward -Infinity(1:w1110) -> (0:w1111:dbl)
          n224 = Bundle("status"=w1100, "code"=w1099, "source"=w1098) -> (w1097:errorcluster)  [unwired: 1 in]
          n225 = Bundle("status"=w1084, "code"=w1082, "source"=w1083) -> (w1080:errorcluster)  [unwired: 1 in]
          n226 = Equal?(x=w1110, y=w1111) -> (x = y?=w1108:bool)
          n227 = while {
            shift-right: [w1147] -> w1069
            shift-left: FALSE -> [w1233]
            tunnel: w1108 -> [w1162]
            tunnel: w1073 -> [w1225]
            tunnel: w1068 -> [w1180]
            tunnel: w1068 -> [w1218]
            tunnel: w1105 -> [w1217]
            shift-right: [w1148] -> w1104
            shift-left: w1107 -> [w1220]
            shift-right: [w1216] -> w1103
            shift-left: w1106 -> [w1219]
            tunnel: [w1215] -> w1102
            tunnel: w1073 -> [w1207]
            tunnel: w1097 -> [w1205]
            tunnel: w1072 -> [w1206]
            tunnel: [w1168] -> w1096
            tunnel: [w1204] -> w1095
            tunnel: w1068 -> [w1167]
            shift-right: [w1165] -> w1087
            shift-left: dbl[][] [] -> [w1160]
            tunnel: [w1196] -> w1092
            tunnel: [w1195] -> w1091
            tunnel: w1088 -> [w1196]
            tunnel: w1093 -> [w1195]
            tunnel: w1073 -> [w1193]
            tunnel: w1081 -> [w1187]
            tunnel: w1080 -> [w1188]
            tunnel: [w1186] -> w1078
            tunnel: [w1185] -> w1079
            shift-right: [w1182] -> w1075
            shift-left: w1077 -> [w1190]
            shift-right: [w1181] -> w1074
            shift-left: w1076 -> [w1197]
            tunnel: w1073 -> [w1179]
            tunnel: w1071 -> [w1159]
            tunnel: w1071 -> [w1163]
            tunnel: [w1159] -> w1070
            tunnel: w1068 -> [w1132]
            shift-right: [w1119] -> w1066
            shift-left: w1067 -> [w1118]
            tunnel: w1065 -> [w1115]
            i -> [w1117]
            stop <- w1121 stop-if-true
            # "Number of measurement loops"
            # "Measurement time (ms)"
            # "Control timing"
            # "Stop measurement cycle"
            # "Set # of cycles"
            # "Write to file"
            # "Add position / Event marks"
            # "Feed graphs"
            # "Get voltage data"
            # "Get time (s) / calculate position of probe"
            # "Control manipulator"
            # "Set graphs and controls"
            # "Stop experiment"
            n228 = Get Date/Time In Seconds() -> (seconds since 1Jan1904=w1116:timestamp)
            n229 = disable-structure shown="Disabled" {
              disable-tunnel: w1206 -> [w1266 _]
              disable-tunnel: w1205 -> [w1265 _]
              disable-tunnel: [w1264 _] -> w1204
              disable-tunnel: [w1263 _] -> w1168
              disable-tunnel: [w1252 _] -> _
              frame Disabled {
                w1250 = 0 ("Index")
                n230 = call-poly <vilib>:"DAQmx Read.vi"("task/channels in"=w1266, "error in"=w1265) -> ("task out"=w1263:refnum<k21>, "data"=w1249:dbl[][], "error out"=w1264:errorcluster)  [unwired: 11 in]
                n231 = Index Array(array=w1249, index (row)=w1250, index (col)=w1250) -> (element=w1258:dbl)
                n232 = Index Array(array=w1249, index (row)=1 ("Index"), index (col)=w1250) -> (element=w1257:dbl)
                n233 = Index Array(array=w1249, index (row)=2 ("Index"), index (col)=w1250) -> (element=w1255:dbl)
                n234 = Index Array(array=w1249, index (row)=3 ("Index"), index (col)=w1250) -> (element=w1256:dbl)
                n235 = Divide(x=w1258, y=-0.0333) -> (x/y=w1253:dbl)
                n236 = Divide(x=w1257, y=-0.0333) -> (x/y=w1254:dbl)
                n237 = Build Array(w1253, w1254, w1255, w1256) -> (w1252:dbl[])
              }
              frame Enabled {
              }
            }
            n238 = Equal To 0?(x=w1117) -> (x = 0?=w1198:bool)
            n239 = Greater Or Equal?(x=w1193, y=2) -> (x >= y?=w1192:bool)
            "E-mark on" <- w1192
            n240 = Subtract(x=w1116, y=w1115) -> (x-y=w1114:dbl)
            n241 = Add(x=w1118, y=1) -> (x+y=w1119:i32)
            n242 = Index Array(array=w1180, index=2) -> (element=w1223:dbl)
            n243 = Multiply(x=w1223, y=100.0) -> (x*y=w1222:dbl)
            n244 = Multiply(x=w1119, y=10) -> (x*y=w1126:i32)
            n245 = Multiply(x=w1114, y=1000.0) -> (x*y=w1122:dbl)
            n246 = case shown="True" w1192 {
              tunnel: [FALSE "Add Mark"] -> w1191
              tunnel: w1190 -> [_ w1507]
              frame False {
              }
              frame True {
                n247 = Array Size(array=w1507) -> (size(s)=w1511:i32)
                n248 = Subtract(x=w1511, y=1) -> (x-y=w1509:i32)
                n249 = Index Array(array=w1507, index=w1509) -> (element=→"String":string)
              }
            }
            n250 = call "Feed-Position-Graph (SubVI).vi"("Array 2"=w1167, "Array"=w1160) -> ("Array 3"=→"Position probe":cluster{dbl[], dbl[]}[])  [unwired: 9 in]
            n251 = Subtract(x=w1122, y=w1126) -> (x-y=w1128:dbl)
            n252 = Index Array(array=w1132, index=2) -> (element=w1138:dbl)
            n253 = Equal?(x=w1179, y=0) -> (x = y?=w1176:bool)
            n254 = Equal?(x=w1117, y=0) -> (x = y?=w1175:bool)
            n255 = Subtract(x=w1222, y=10.0) -> (x-y=w1230:dbl)
            n256 = Subtract(x=w1222, y=20.0) -> (x-y=w1229:dbl)
            n257 = Equal?(x=w1225, y=0) -> (x = y?=w1154:bool)
            n258 = And(x=w1176, y=w1175) -> (x .and. y?=w1174:bool)
            n259 = Multiply(x=w1128, y=-1.0) -> (x*y=w1125:dbl)
            n260 = Build Array(0, 10, w1229, w1230) -> (w1113:dbl[])
            n261 = Multiply(x=w1138, y=100.0) -> (x*y=w1134:dbl)
            n262 = case shown="False" w1154 {
              tunnel: [w1610 w1628] -> w1153
              tunnel: w1113 -> [w1609 w1627]
              tunnel: w1117 -> [w1608 w1626]
              frame False {
                n263 = for {
                  tunnel: w1609 -> [w1617] mode=indexing
                  tunnel: w1608 -> [w1618]
                  shift-right: [w1615] -> w1610
                  shift-left: 0 -> [w1616]
                  i -> [w1613]
                  n264 = Equal?(x=w1617, y=w1618) -> (x = y?=w1614:bool)
                  n265 = case shown="True" w1614 {
                    tunnel: w1613 -> [_ w1621]
                    tunnel: [0 w1620] -> w1612
                    frame False {
                    }
                    frame True {
                      n266 = case shown="3" w1621 {
                        tunnel: [1 2 3 5] -> w1620
                        frame 0, Default {
                        }
                        frame 1 {
                        }
                        frame 2 {
                        }
                        frame 3 {
                        }
                      }
                    }
                  }
                  n267 = Add(x=w1616, y=w1612) -> (x+y=w1615:i32)
                }
              }
              frame True {
                n268 = for {
                  tunnel: w1627 -> [w1635] mode=indexing
                  tunnel: w1626 -> [w1636]
                  shift-right: [w1633] -> w1628
                  shift-left: 0 -> [w1634]
                  i -> [w1632]
                  n269 = Equal?(x=w1635, y=w1636) -> (x = y?=w1630:bool)
                  n270 = case shown="True" w1630 {
                    tunnel: w1632 -> [_ w1638]
                    tunnel: [0 w1639] -> w1631
                    frame False {
                    }
                    frame True {
                      n271 = case shown="3" w1638 {
                        tunnel: [0 0 3 4] -> w1639
                        frame 0, Default {
                        }
                        frame 1 {
                        }
                        frame 2 {
                        }
                        frame 3 {
                        }
                      }
                    }
                  }
                  n272 = Add(x=w1634, y=w1631) -> (x+y=w1633:i32)
                }
              }
            }
            n273 = Add(x=1 ("y"), y=w1117) -> (x+y=w1135:i32)
            n274 = Index Array(array=w1180, index=3 ("Index")) -> (element=w1213:dbl)
            n275 = Equal?(x=w1134, y=w1135) -> (x = y?=w1121:bool)
            n276 = Index Array(array=w1180, index=0 ("Index")) -> (element=w1209:dbl)
            n277 = Divide(x=w1213, y=10.0) -> (x/y=w1208:dbl)
            n278 = Greater?(x=w1208, y=w1117) -> (0:w1211:bool)
            n279 = case shown="True" w1211 {
              tunnel: w1209 -> [w1582 w1588]
              tunnel: w1117 -> [_ w1590]
              tunnel: w1162 -> [w1584 w1593]
              tunnel: w1208 -> [_ w1592]
              tunnel: [w1583 w1589] -> w1199
              tunnel: w1207 -> [_ w1587]
              frame False {
                n280 = case shown="False" w1584 {
                  tunnel: [w1585 0.0] -> w1583
                  tunnel: w1582 -> [w1585 _]
                  frame False {
                  }
                  frame True {
                  }
                }
              }
              frame True {
                n281 = Divide(x=w1588, y=w1592) -> (x/y=w1591:dbl)
                n282 = case shown="True" w1593 {
                  tunnel: w1590 -> [w1596 w1600]
                  tunnel: w1591 -> [w1595 w1604]
                  tunnel: [w1594 w1598] -> w1589
                  tunnel: w1588 -> [_ w1603]
                  tunnel: w1587 -> [_ w1597]
                  frame False {
                    n283 = Multiply(x=w1595, y=w1596) -> (x*y=w1594:dbl)
                  }
                  frame True {
                    n284 = Multiply(x=w1604, y=w1600) -> (x*y=w1605:dbl)
                    n285 = Equal?(x=w1597, y=0) -> (x = y?=w1602:bool)
                    n286 = Subtract(x=w1603, y=w1605) -> (x-y=w1599:dbl)
                    n287 = case shown="True" w1602 {
                      tunnel: [w1606 0.0] -> w1598
                      tunnel: w1599 -> [w1606 _]
                      frame False {
                      }
                      frame True {
                      }
                    }
                  }
                }
              }
            }
            n288 = case shown="\"SISE chan #1\", Default" "?" {
              selector: "?" -> [w1451 w1461 w1469 w1477]
              tunnel: w1167 -> [w1456 w1463 w1473 w1480]
              tunnel: w1160 -> [w1457 w1464 w1472 w1481]
              tunnel: w1163 -> [w1453 w1460 w1467 w1476]
              tunnel: "Start fit (% of rec. period)" -> [w1455 w1462 w1471 w1479]
              frame "SISE chan #1", Default {
                n289 = Index Array(array=w1453, index=w1451) -> (element=w1452:bool)
                n290 = call "Feed-SISE-Probe-Graph.vi"("Boolesch"=w1452, "Numerisch"=2, "Array 2"=w1457, "Array"=w1456, "Start fit (% of rec. period)"=w1455) -> ("Array 3"=→"Vprobe SISE 1":cluster{dbl[], dbl[]}[])  [unwired: 6 in]
              }
              frame "SISE chan #2" {
                n291 = Index Array(array=w1460, index=w1461) -> (element=w1459:bool)
                n292 = call "Feed-SISE-Probe-Graph.vi"("Boolesch"=w1459, "Numerisch"=3, "Array 2"=w1464, "Array"=w1463, "Start fit (% of rec. period)"=w1462) -> ("Array 3"=→"Vprobe SISE 2":cluster{dbl[], dbl[]}[])  [unwired: 6 in]
              }
              frame "V chan #1" {
                n293 = Index Array(array=w1467, index=w1469) -> (element=w1468:bool)
                n294 = call "Feed-V-Probe-Graph.vi"("Boolesch"=w1468, "Numerisch"=4, "Array 2"=w1472, "Array"=w1473, "Start fit (% of rec. period)"=w1471) -> ("Array 3"=→"Vprobe V 1":cluster{dbl[], dbl[]}[])  [unwired: 6 in]
              }
              frame "V chan #2" {
                n295 = Index Array(array=w1476, index=w1477) -> (element=w1475:bool)
                n296 = call "Feed-V-Probe-Graph.vi"("Boolesch"=w1475, "Numerisch"=5, "Array 2"=w1481, "Array"=w1480, "Start fit (% of rec. period)"=w1479) -> ("Array 3"=→"Vprobe V 2":cluster{dbl[], dbl[]}[])  [unwired: 6 in]
              }
            }
            n297 = disable-structure shown="Disabled" {
              disable-tunnel: w1220 -> [w1275 _]
              disable-tunnel: w1219 -> [w1274 _]
              disable-tunnel: w1218 -> [w1273 _]
              disable-tunnel: w1217 -> [w1272 _]
              disable-tunnel: [w1271 _] -> w1216
              disable-tunnel: [w1270 _] -> w1215
              disable-tunnel: w1162 -> [w1269 _]
              disable-tunnel: w1153 -> [w1268 _]
              disable-tunnel: [w1267 _] -> w1148
              frame Disabled {
                n298 = case shown="1" w1268 {
                  tunnel: w1272 -> [w1276 w1289 w1333 w1340 w1352 w1399]
                  tunnel: w1274 -> [w1278 w1296 w1336 w1339 w1351 w1398]
                  tunnel: [w1278 w1296 w1336 w1339 w1350 w1397] -> w1271
                  tunnel: w1273 -> [_ w1295 _ _ _ _]
                  tunnel: w1269 -> [_ w1283 _ _ w1344 w1391]
                  tunnel: w1275 -> [w1277 w1282 w1332 w1338 w1347 w1394]
                  tunnel: [w1277 w1282 w1332 w1338 w1348 w1395] -> w1267
                  tunnel: [w1276 w1281 w1331 w1337 w1345 w1392] -> w1270
                  frame 0, Default {
                  }
                  frame 1 {
                    n299 = local read "left"() -> (w1280:bool)
                    n300 = Index Array(array=w1295, index=0) -> (element=w1297:dbl)
                    n301 = Index Array(array=w1295, index=1) -> (element=w1288:dbl)
                    n302 = Cosine(x=w1288) -> (cos(x)=w1287:dbl)
                    n303 = Sine(x=w1288) -> (sin(x)=w1286:dbl)
                    n304 = case shown="False" w1280 {
                      tunnel: [10.0 -10.0] -> w1279
                      frame False {
                      }
                      frame True {
                      }
                    }
                    n305 = Multiply(x=w1297, y=w1287) -> (x*y=w1294:dbl)
                    n306 = Multiply(x=w1297, y=w1286) -> (x*y=w1293:dbl)
                    n307 = Multiply(x=w1294, y=w1279) -> (x*y=w1291:dbl)
                    n308 = Multiply(x=w1293, y=10.0) -> (x*y=w1292:dbl)
                    n309 = for {
                      tunnel: w1296 -> [w1311] mode=indexing
                      tunnel: w1291 -> [w1313]
                      tunnel: w1292 -> [w1312]
                      shift-right: [w1307] -> w1285
                      shift-left: "ABS " -> [w1309]
                      tunnel: w1283 -> [w1302]
                      i -> [w1304]
                      n310 = case shown="True" w1302 {
                        tunnel: w1304 -> [w1314 _]
                        tunnel: [w1314 1] -> w1303
                        frame False {
                        }
                        frame True {
                        }
                      }
                      n311 = case shown="1" w1303 {
                        tunnel: w1313 -> [w1325 _ _]
                        tunnel: w1312 -> [_ _ w1329]
                        tunnel: w1311 -> [w1326 w1327 w1330]
                        tunnel: [w1324 w1327 w1328] -> w1310
                        frame 0, Default {
                          n312 = Add(x=w1326, y=w1325) -> (x+y=w1324:dbl)
                        }
                        frame 1 {
                        }
                        frame 2 {
                          n313 = Add(x=w1330, y=w1329) -> (x+y=w1328:dbl)
                        }
                      }
                      n314 = Number To Decimal String(number=w1310) -> (decimal integer string=w1308:string)  [unwired: 1 in]
                      n315 = Equal?(x=2, y=w1304) -> (x = y?=w1305:bool)
                      n316 = case shown="True" w1305 {
                        tunnel: w1309 -> [w1319 w1323]
                        tunnel: w1308 -> [w1318 w1321]
                        tunnel: [w1316 w1322] -> w1307
                        frame False {
                          n317 = Concatenate Strings(w1319, w1318, "\t") -> (w1316:string)
                        }
                        frame True {
                          n318 = Concatenate Strings(w1323, w1321, "\r\n") -> (w1322:string)
                        }
                      }
                    }
                    n319 = VISA Write(VISA resource name=w1289, write buffer=w1285) -> (VISA resource name out=w1281:refnum<visa-resource-name>)  [unwired: 1 in, 2 out]
                  }
                  frame 2 {
                    n320 = property class="Instr"(reference=w1333) -> (reference out=w1334:refnum<visa-resource-name>, "Bytes at Port"=w1335:u32)  [unwired: 1 in, 1 out]
                    n321 = VISA Read(VISA resource name=w1334, byte count=w1335) -> (VISA resource name out=w1331:refnum<visa-resource-name>)  [unwired: 1 in, 3 out]
                  }
                  frame 3 {
                    n322 = Concatenate Strings("POS", "\r\n") -> (w1343:string)
                    n323 = VISA Write(VISA resource name=w1340, write buffer=w1343) -> (VISA resource name out=w1337:refnum<visa-resource-name>)  [unwired: 1 in, 2 out]
                  }
                  frame 4 {
                    n324 = property class="Instr"(reference=w1352) -> (reference out=w1354:refnum<visa-resource-name>, "Bytes at Port"=w1353:u32)  [unwired: 1 in, 1 out]
                    n325 = VISA Read(VISA resource name=w1354, byte count=w1353) -> (VISA resource name out=w1346:refnum<visa-resource-name>, read buffer=w1349:string)  [unwired: 1 in, 2 out]
                    n326 = case shown="True" w1344 {
                      tunnel: w1351 -> [w1370 w1389]
                      tunnel: [w1370 w1388] -> w1350
                      tunnel: w1349 -> [w1359 w1374]
                      tunnel: [w1364 w1383] -> w1348
                      tunnel: w1347 -> [w1363 w1382]
                      tunnel: w1346 -> [w1355 w1373]
                      tunnel: [w1355 w1373] -> w1345
                      frame False {
                        n327 = Match Pattern(string=w1363, regular expression="P0:") -> (match substring=w1368:string, after substring=w1367:string)  [unwired: 1 in, 2 out]
                        n328 = String Length(string=w1359) -> (length=w1362:i32)
                        n329 = Match Pattern(string=w1367, regular expression="P1:") -> (before substring=w1356:string, match substring=w1369:string)  [unwired: 1 in, 2 out]
                        n330 = Subtract(x=w1362, y=1) -> (x-y=w1360:i32)
                        n331 = String Subset(string=w1359, length (rest)=w1360) -> (substring=w1358:string)  [unwired: 1 in]
                        n332 = Concatenate Strings(w1368, w1356, w1369, w1358, "\t") -> (w1364:string)
                      }
                      frame True {
                        n333 = Match Pattern(string=w1382, regular expression="P0:") -> (match substring=w1384:string, after substring=w1386:string)  [unwired: 1 in, 2 out]
                        n334 = String Length(string=w1374) -> (length=w1381:i32)
                        n335 = Subtract(x=w1381, y=1) -> (x-y=w1379:i32)
                        n336 = Match Pattern(string=w1386, regular expression="P1:") -> (match substring=w1376:string, after substring=w1377:string)  [unwired: 1 in, 2 out]
                        n337 = String Subset(string=w1374, length (rest)=w1379) -> (substring=w1378:string)  [unwired: 1 in]
                        n338 = Concatenate Strings(w1384, w1378, "\t", w1376, w1377) -> (w1383:string)
                        n339 = call "GetAxisValuesI (SubVI).vi"("read buffer"=w1374) -> ("Array"=w1371:dbl[])  [unwired: 10 in]
                        n340 = Replace Array Subset(array=w1389, new element=w1371, index=0 ("Index")) -> (w1388:dbl[])
                      }
                    }
                  }
                  frame 5 {
                    n341 = property class="Instr"(reference=w1399) -> (reference out=w1401:refnum<visa-resource-name>, "Bytes at Port"=w1400:u32)  [unwired: 1 in, 1 out]
                    n342 = VISA Read(VISA resource name=w1401, byte count=w1400) -> (VISA resource name out=w1393:refnum<visa-resource-name>, read buffer=w1396:string)  [unwired: 1 in, 2 out]
                    n343 = case shown="True" w1391 {
                      tunnel: w1398 -> [w1417 w1436]
                      tunnel: [w1417 w1435] -> w1397
                      tunnel: w1396 -> [w1406 w1421]
                      tunnel: [w1411 w1430] -> w1395
                      tunnel: w1394 -> [w1410 w1429]
                      tunnel: w1393 -> [w1402 w1419]
                      tunnel: [w1402 w1418] -> w1392
                      tunnel: "Enable change position 0" -> [_ w1420]
                      frame False {
                        n344 = Match Pattern(string=w1410, regular expression="P0:") -> (match substring=w1415:string, after substring=w1414:string)  [unwired: 1 in, 2 out]
                        n345 = String Length(string=w1406) -> (length=w1409:i32)
                        n346 = Match Pattern(string=w1414, regular expression="P1:") -> (before substring=w1403:string, match substring=w1416:string)  [unwired: 1 in, 2 out]
                        n347 = Subtract(x=w1409, y=1) -> (x-y=w1407:i32)
                        n348 = String Subset(string=w1406, length (rest)=w1407) -> (substring=w1405:string)  [unwired: 1 in]
                        n349 = Concatenate Strings(w1415, w1403, w1416, w1405, "\t") -> (w1411:string)
                      }
                      frame True {
                        n350 = Match Pattern(string=w1429, regular expression="P0:") -> (match substring=w1431:string, after substring=w1433:string)  [unwired: 1 in, 2 out]
                        n351 = String Length(string=w1421) -> (length=w1428:i32)
                        n352 = Subtract(x=w1428, y=1) -> (x-y=w1426:i32)
                        n353 = Match Pattern(string=w1433, regular expression="P1:") -> (match substring=w1423:string, after substring=w1424:string)  [unwired: 1 in, 2 out]
                        n354 = String Subset(string=w1421, length (rest)=w1426) -> (substring=w1425:string)  [unwired: 1 in]
                        n355 = case shown="False" w1420 {
                          tunnel: w1436 -> [w1438 w1444]
                          tunnel: [w1438 w1443] -> w1435
                          tunnel: w1421 -> [_ w1442]
                          tunnel: w1419 -> [w1437 w1439]
                          tunnel: [w1437 w1439] -> w1418
                          frame False {
                          }
                          frame True {
                            n356 = call "GetAxisValuesI (SubVI).vi"("read buffer"=w1442) -> ("Array"=w1440:dbl[])  [unwired: 10 in]
                            n357 = Replace Array Subset(array=w1444, new element=w1440, index=0 ("Index")) -> (w1443:dbl[])
                          }
                        }
                        n358 = Concatenate Strings(w1431, w1425, "\t", w1423, w1424) -> (w1430:string)
                      }
                    }
                  }
                }
              }
              frame Enabled {
              }
            }
            n359 = case shown="True" w1198 {
              tunnel: w1148 -> [_ w1533]
              tunnel: [w1517 w1533] -> w1183
              tunnel: w1191 -> [w1518 _]
              tunnel: w1190 -> [w1513 w1542]
              tunnel: w1114 -> [w1516 w1541]
              tunnel: [w1515 w1533] -> w1181
              tunnel: w1197 -> [w1515 w1534]
              tunnel: [w1514 w1540] -> w1182
              frame False {
                n360 = case shown="True" w1518 {
                  tunnel: ["" "Event Mark"] -> w1517
                  tunnel: w1516 -> [_ w1532]
                  tunnel: w1513 -> [w1520 w1525]
                  tunnel: [w1520 w1526] -> w1514
                  frame False {
                  }
                  frame True {
                    n361 = Divide(x=w1532, y=60.0) -> (x/y=w1530:dbl)
                    n362 = Number To Fractional String(number=w1530, precision (6)=i16 2 ("Genauigkeit (6)")) -> (F-format string=w1528:string)  [unwired: 2 in]
                    n363 = Concatenate Strings(w1528, " min: ", "\t", "Event Mark", "\t") -> (w1524:string)
                    n364 = Insert Into Array(array=w1525, new element=w1524) -> (w1526:string[])  [unwired: 1 in]
                  }
                }
              }
              frame True {
                n365 = Match Pattern(string=w1533, regular expression="P1:") -> (before substring=w1537:string)  [unwired: 1 in, 3 out]
                n366 = Match Pattern(string=w1534, regular expression="P1:") -> (before substring=w1535:string)  [unwired: 1 in, 3 out]
                n367 = Not Equal?(x=w1537, y=w1535) -> (x != y?=w1539:bool)
                n368 = case shown="True" w1539 {
                  tunnel: w1542 -> [w1543 w1565]
                  tunnel: [w1543 w1566] -> w1540
                  tunnel: w1533 -> [_ w1554]
                  tunnel: w1534 -> [_ w1553]
                  tunnel: w1541 -> [_ w1551]
                  frame False {
                  }
                  frame True {
                    n369 = Divide(x=w1551, y=60.0) -> (x/y=w1549:dbl)
                    n370 = Match Pattern(string=w1554, regular expression="P0:") -> (after substring=w1564:string)  [unwired: 1 in, 3 out]
                    n371 = Number To Fractional String(number=w1549, precision (6)=i16 2) -> (F-format string=w1545:string)  [unwired: 2 in]
                    n372 = Match Pattern(string=w1553, regular expression="P0:") -> (after substring=w1559:string)  [unwired: 1 in, 3 out]
                    n373 = Match Pattern(string=w1564, regular expression="P1:") -> (before substring=w1563:string)  [unwired: 1 in, 3 out]
                    n374 = Match Pattern(string=w1559, regular expression="P1:") -> (before substring=w1558:string)  [unwired: 1 in, 3 out]
                    n375 = Concatenate Strings(w1545, "\t", "min: Move ") -> (w1548:string)
                    n376 = call "GetAxisValuesII (SubVI).vi"("read buffer"=w1563) -> ("Array"=w1560:dbl[])  [unwired: 10 in]
                    n377 = call "GetAxisValuesII (SubVI).vi"("read buffer"=w1558) -> ("Array"=w1555:dbl[])  [unwired: 10 in]
                    n378 = for {
                      tunnel: w1560 -> [w1576] mode=indexing
                      tunnel: w1555 -> [w1575] mode=indexing
                      shift-right: [w1577] -> w1546
                      shift-left: w1548 -> [w1578]
                      i -> [w1573]
                      n379 = Subtract(x=w1576, y=w1575) -> (x-y=w1570:dbl)
                      n380 = Divide(x=w1570, y=10.0) -> (x/y=w1572:dbl)
                      n381 = case shown="0, Default" w1573 {
                        tunnel: ["X " "Y " "Z "] -> w1569
                        frame 0, Default {
                        }
                        frame 1 {
                        }
                        frame 2 {
                        }
                      }
                      n382 = Number To Fractional String(number=w1572, precision (6)=i16 2 ("Genauigkeit (6)")) -> (F-format string=w1568:string)  [unwired: 2 in]
                      n383 = Concatenate Strings(w1578, w1569, w1568, "\t") -> (w1577:string)
                    }
                    n384 = Insert Into Array(array=w1565, new element=w1546) -> (w1566:string[])  [unwired: 1 in]
                  }
                }
              }
            }
            n385 = for {
              tunnel: w1113 -> [w1238] mode=indexing
              tunnel: w1117 -> [w1239]
              shift-right: [w1235] -> w1123
              shift-left: FALSE -> [w1236]
              n386 = Equal?(x=w1238, y=w1239) -> (x = y?=w1237:bool)
              n387 = case shown="False" w1237 {
                tunnel: w1236 -> [w1240 _]
                tunnel: [w1240 TRUE] -> w1235
                frame False {
                }
                frame True {
                }
              }
            }
            n388 = case shown="True" w1174 {
              frame False {
              }
              frame True {
                n389 = Build Array(0.0, 0.0) -> (w1500:dbl[])
                n390 = Build Array(0.0, 30.0) -> (w1501:dbl[])
                n391 = Bundle(w1501, w1500) -> (w1499:cluster{dbl[], dbl[]})  [unwired: 1 in]
                n392 = Build Array(w1499, w1499, w1499, w1499) -> (w1497:cluster{dbl[], dbl[]}[])
                n393 = local write "dV-SISE channel 1"(w1497) -> ()
                n394 = local write "deltaV SISE 1"(w1497) -> ()
                n395 = local write "deltaV SISE 2"(w1497) -> ()
                n396 = local write "V-SISE channel 1"(w1497) -> ()
                n397 = local write "Enable change position 0"(FALSE) -> ()
                n398 = local write "V-SISE channel 2"(w1497) -> ()
                n399 = local write "dV-SISE channel 2"(w1497) -> ()
                n400 = local write "Voltage channel 1"(w1497) -> ()
                n401 = local write "Voltage channel 2"(w1497) -> ()
              }
            }
            n402 = case shown="False" w1123 {
              tunnel: w1125 -> [w1244 _]
              tunnel: [w1243 10.0] -> w1120
              frame False {
                n403 = Less?(x=w1244, y=7.0) -> (x < y?=w1242:bool)
                n404 = case shown="False" w1242 {
                  tunnel: w1244 -> [w1246 _]
                  tunnel: [w1246 7.0] -> w1243
                  frame False {
                  }
                  frame True {
                  }
                }
              }
              frame True {
              }
            }
            n405 = call "EsingleGenerator.vi"("Numeric in"=w1117, "Boolean"=w1162) -> ("Numeric out"=w1142:dbl)  [unwired: 9 in]
            n406 = Build Array(w1114, w1199) -> (w1149:dbl[])
            n407 = Wait (ms)(milliseconds to wait=w1120) -> ()  [unwired: 1 out]
            n408 = Multiply(x=w1142, y="V SISE\nch #1") -> (x*y=w1145:dbl)
            n409 = Multiply(x=w1142, y="V SISE\nch #2") -> (x*y=w1144:dbl)
            n410 = Random Number (0-1)() -> (number: 0 to 1=w1173:dbl)
            n411 = Random Number (0-1)() -> (number: 0 to 1=w1203:dbl)
            n412 = Add(x=w1144, y=8.0) -> (x+y=w1172:dbl)
            n413 = Add(x=w1145, y=6.0) -> (x+y=w1202:dbl)
            n414 = Add(x=w1172, y=w1173) -> (x+y=w1169:dbl)
            n415 = Add(x=w1202, y=w1203) -> (x+y=w1170:dbl)
            n416 = case shown="False" "Stop measurent" {
              tunnel: [w1644 TRUE] -> w1147
              tunnel: w1233 -> [w1644 _]
              frame False {
              }
              frame True {
              }
            }
            "Stop recording" <- w1147
            n417 = Build Array(w1170, w1169, "Vch #1", "Vch\n#2") -> (w1139:dbl[])
            n418 = for {
              tunnel: w1139 -> [w1484] mode=indexing
              tunnel: w1159 -> [w1487] mode=indexing
              shift-right: [w1485] -> w1158
              shift-left: dbl[] [] -> [w1486]
              shift-right: [w1482] -> w1150
              shift-left: dbl[] [] -> [w1483]
              n419 = case shown="False" w1487 {
                tunnel: w1486 -> [w1491 w1496]
                tunnel: [w1491 w1495] -> w1485
                tunnel: w1484 -> [_ w1492]
                tunnel: w1483 -> [w1490 w1494]
                tunnel: [w1489 w1493] -> w1482
                frame False {
                  n420 = Insert Into Array(array=w1490, new element=0.0 ("Neues Element/Teil-Array")) -> (w1489:dbl[])  [unwired: 1 in]
                }
                frame True {
                  n421 = Insert Into Array(array=w1496, new element=w1492) -> (w1495:dbl[])  [unwired: 1 in]
                  n422 = Insert Into Array(array=w1494, new element=w1492) -> (w1493:dbl[])  [unwired: 1 in]
                }
              }
            }
            n423 = Insert Into Array(array=w1149, new element=w1150) -> (w1151:dbl[])  [unwired: 1 in]
            n424 = Insert Into Array(array=w1149, new element=w1158) -> (w1156:dbl[])  [unwired: 1 in]
            n425 = for {
              tunnel: w1156 -> [w1447] mode=indexing
              shift-right: [w1446] -> w1155
              shift-left: "" -> [w1448]
              n426 = Number To Fractional String(number=w1447) -> (F-format string=w1449:string)  [unwired: 3 in]
              n427 = Concatenate Strings(w1448, w1449, "\t") -> (w1446:string)
            }
            n428 = Insert Into Array(array=w1160, new element=w1151) -> (w1165:dbl[][])  [unwired: 2 in]
            n429 = Concatenate Strings(w1155, w1183, "\r\n") -> (w1184:string)
            n430 = Write to Text File(file (use dialog)=w1187, text=w1184, error in=w1188) -> (refnum out=w1186:refnum<file>, error out=w1185:errorcluster)  [unwired: 1 in, 1 out]
          }
          "Stop recording 2" <- w1069
          n431 = Bundle(w1075, w1087) -> (w1086:cluster{string[], dbl[][]})  [unwired: 1 in]
          n432 = Enqueue Element(queue=w1092, element=w1086, error in (no error)=w1091) -> (queue out=w1090:refnum<queue>, error out=w1089:errorcluster)  [unwired: 1 in, 1 out]
        }
        n433 = while {
          tunnel: w551 -> [w631]
          tunnel: w545 -> [w611]
          shift-right: [w583] -> _
          shift-left: w546 -> [w626]
          shift-right: [w600] -> _
          shift-left: dbl[][] [] -> [w601]
          shift-right: [w602] -> _
          shift-left: string[] ["Time, Event mark"] -> [w603]
          tunnel: w525 -> [w573]
          i -> [w582]
          stop <- w627 stop-if-true
          # "Replace time axis"
          # "Calculate average values"
          # "Determine dV"
          # "Combine traces for regression"
          n434 = local read "Stop recording"() -> (w628:bool)
          n435 = Dequeue Element(queue=w631) -> (element=w606:cluster{string[], dbl[][]}, error out=w630:errorcluster)  [unwired: 2 in, 2 out]
          n436 = local read "Start fit (% of rec. period)"() -> (w615:dbl)
          n437 = Greater Or Equal?(x=w582, y=2) -> (x >= y?=w593:bool)
          n438 = Unbundle By Name(w630) -> ("status"=w629:bool)
          n439 = Or(x=w629, y=w628) -> (x .or. y?=w627:bool)
          n440 = Unbundle(w606) -> (w604:string[], w605:dbl[][])
          n441 = Multiply(x=w611, y=w615) -> (x*y=w596:dbl)
          n442 = Multiply(x=w611, y=100.0) -> (x*y=w597:dbl)
          n443 = Multiply(x=w611, y=100.0) -> (x*y=w624:dbl)
          n444 = Multiply(x=w611, y=200.0) -> (x*y=w623:dbl)
          n445 = Array Subset(array=w626, index (row)=w624, length (row)=w623) -> (w620:dbl[][])  [unwired: 2 in]
          n446 = Delete From Array(array=w605, index (col)=1 ("Deaktivierter Index (Spalte)")) -> (array with subset deleted=w619:dbl[][])  [unwired: 2 in, 1 out]
          n447 = Insert Into Array(array=w620, new element=w619) -> (w583:dbl[][])  [unwired: 2 in]
          n448 = local read "Start fit (% of rec. period)"() -> (w612:dbl)
          n449 = Multiply(x=w611, y=w612) -> (x*y=w609:dbl)
          n450 = Multiply(x=w611, y=100.0) -> (x*y=w608:dbl)
          n451 = Add(x=w609, y=w608) -> (x+y=w610:dbl)
          n452 = Subtract(x=w608, y=w609) -> (x-y=w598:dbl)
          n453 = Array Subset(array=w583, index (row)=w610, length (row)=w598) -> (w585:dbl[][])  [unwired: 2 in]
          n454 = Transpose 2D Array(2D array=w585) -> (transposed array=w584:dbl[][])
          n455 = for {
            tunnel: w584 -> [w720] mode=indexing
            shift-right: [w719] -> w588
            shift-left: dbl[] [] -> [w718]
            n456 = Add Array Elements(numeric array=w720) -> (sum=w721:dbl)
            n457 = Array Size(array=w720) -> (size(s)=w722:i32)
            n458 = Divide(x=w721, y=w722) -> (x/y=w717:dbl)
            n459 = Insert Into Array(array=w718, new element=w717) -> (w719:dbl[])  [unwired: 1 in]
          }
          n460 = Index Array(array=w583, index (col)=0 ("Deaktivierter Index (Spalte)")) -> (element=w592:dbl[])  [unwired: 1 in]
          n461 = Index Array(array=w588, index=0 ("Index (Spalte)")) -> (element=w590:dbl)
          n462 = for {
            tunnel: w590 -> [w1061]
            shift-right: [w1064] -> w616
            shift-left: dbl[] [] -> [w1063]
            tunnel: w592 -> [w1060] mode=indexing
            n463 = Subtract(x=w1060, y=w1061) -> (x-y=w1062:dbl)
            n464 = Insert Into Array(array=w1063, new element=w1062) -> (w1064:dbl[])  [unwired: 1 in]
          }
          n465 = Replace Array Subset(array=w583, new element=w616, index (col)=0 ("Deaktivierter Index (Spalte)")) -> (w589:dbl[][])  [unwired: 1 in]
          n466 = for {
            N: 2 -> [_]
            tunnel: w589 -> [w647]
            tunnel: w597 -> [w646]
            tunnel: w596 -> [w645]
            tunnel: w593 -> [w641]
            tunnel: w582 -> [w639]
            shift-right: [w638] -> w586
            shift-left: dbl[] [] -> [w637]
            i -> [w644]
            n467 = flat-sequence {
              tunnel: w647 -> [w658]
              tunnel: w645 -> [w659]
              tunnel: w646 -> [w666]
              tunnel: [w663] -> w649
              tunnel: [w660] -> w648
              tunnel: w640 -> [w654]
              tunnel: w649 -> [w690]
              tunnel: w648 -> [w696]
              tunnel: w639 -> [w691]
              tunnel: [w679] -> w636
              tunnel: [w678] -> w642
              frame #0 {
                n468 = Subtract(x=w666, y=w659) -> (x-y=w672:dbl)
                n469 = Multiply(x=w666, y=2.0) -> (x*y=w669:dbl)
                n470 = Add(x=w659, y=w669) -> (x+y=w677:dbl)
                n471 = Add(x=w659, y=w666) -> (x+y=w676:dbl)
                n472 = Array Subset(array=w658, index (row)=w659, length (row)=w672) -> (w674:dbl[][])  [unwired: 2 in]
                n473 = Array Subset(array=w658, index (row)=w677, length (row)=w672) -> (w675:dbl[][])  [unwired: 2 in]
                n474 = Array Subset(array=w658, index (row)=w676, length (row)=w672) -> (w667:dbl[][])  [unwired: 2 in]
                n475 = Insert Into Array(array=w674, new element=w675) -> (w670:dbl[][])  [unwired: 2 in]
                n476 = Index Array(array=w667, index (col)=w654) -> (element=w657:dbl[])  [unwired: 1 in]
                n477 = Index Array(array=w670, index (col)=0 ("disabled index (col)")) -> (element=w665:dbl[])  [unwired: 1 in]
                n478 = Index Array(array=w667, index (col)=0 ("disabled index (col)")) -> (element=w656:dbl[])  [unwired: 1 in]
                n479 = Index Array(array=w670, index (col)=w654) -> (element=w664:dbl[])  [unwired: 1 in]
                n480 = call <vilib>:"Linear Fit.vi"("Y"=w664, "X"=w665) -> ("Best Linear Fit"=w655:dbl[], "slope"=w662:dbl, "intercept"=w661:dbl)  [unwired: 9 in, 2 out]
                n481 = Build Array(w662, w661) -> (w660:dbl[])
                n482 = Bundle(w665, w664, "Best Linear Fit"=w655, w656, w657) -> (w663:T8)  [unwired: 1 in]
              }
              frame #1 {
                n483 = Unbundle(w690) -> (w701:dbl[], w702:dbl[])  [unwired: 3 out]
                n484 = Divide(x=w691, y=2 ("x")) -> (x/y=w692:dbl)
                n485 = Index Array(array=w696, index=0 ("Index")) -> (element=w703:dbl)
                n486 = Index Array(array=w696, index=1 ("Index")) -> (element=w695:dbl)
                n487 = Unbundle(w690) -> (w687:dbl[], w689:dbl[], "Best Linear Fit"=w686:dbl[], w685:dbl[], w683:dbl[])
                n488 = Round To Nearest(number=w692) -> (nearest integer value=w693:dbl)
                n489 = Absolute Value(x=w703) -> (abs(x)=w708:dbl)
                n490 = Equal?(x=w693, y=w692) -> (x = y?=w698:bool)
                n491 = Divide(x=w708, y=1000.0) -> (x/y=w710:dbl)
                n492 = Bundle(w687, w689) -> (w688:cluster{dbl[], dbl[]})  [unwired: 1 in]
                n493 = Bundle(w687, "Best Linear Fit"=w686) -> (w682:cluster{dbl[], "Best Linear Fit":dbl[]})  [unwired: 1 in]
                n494 = Bundle(w685, w683) -> (w680:cluster{dbl[], dbl[]})  [unwired: 1 in]
                n495 = Subtract(x=w703, y=w710) -> (x-y=w707:dbl)
                n496 = Add(x=w703, y=w710) -> (x+y=w706:dbl)
                n497 = Bundle(w707, w706, -inf, inf) -> (w705:cluster{dbl, dbl, dbl, dbl})  [unwired: 1 in]
                n498 = call <vilib>:"Linear Fit.vi"("Y"=w702, "X"=w701, "parameter bounds"=w705) -> ("Best Linear Fit"=w684:dbl[], "intercept"=w694:dbl)  [unwired: 8 in, 3 out]
                n499 = Subtract(x=w695, y=w694) -> (x-y=w699:dbl)
                n500 = Bundle(w685, "Best Linear Fit"=w684) -> (w681:cluster{dbl[], "Best Linear Fit":dbl[]})  [unwired: 1 in]
                n501 = case shown="True" w698 {
                  tunnel: w699 -> [w713 w715]
                  tunnel: [w713 w716] -> w679
                  frame False {
                  }
                  frame True {
                    n502 = Multiply(x=-1.0, y=w715) -> (x*y=w716:dbl)
                  }
                }
                n503 = Build Array(w688, w682, w681, w680) -> (w678:cluster{dbl[], "Best Linear Fit":dbl[]}[])
              }
            }
            n504 = Add(x=1, y=w644) -> (x+y=w640:i32)
            n505 = case shown="True" w641 {
              tunnel: w642 -> [_ w651]
              tunnel: w640 -> [_ w650]
              frame False {
              }
              frame True {
                n506 = case shown="0, Default" w650 {
                  tunnel: w651 -> [_ w652 w653]
                  frame 0, Default {
                  }
                  frame 1 {
                    "deltaV SISE 1" <- w652
                  }
                  frame 2 {
                    "deltaV SISE 2" <- w653
                  }
                }
              }
            }
            n507 = Insert Into Array(array=w637, new element=w636) -> (w638:dbl[])  [unwired: 1 in]
          }
          n508 = Insert Into Array(array=w588, index=3 ("Index"), new element=w586) -> (w575:dbl[])
          n509 = Index Array(array=w575, index=0 ("Index")) -> (element=w577:dbl)
          n510 = Divide(x=w577, y=60.0) -> (x/y=w576:dbl)
          n511 = Replace Array Subset(array=w575, new element=w576, index=0 ("Index")) -> (w574:dbl[])
          n512 = case shown="True" w593 {
            tunnel: w601 -> [w632 w635]
            tunnel: [w632 w634] -> w600
            tunnel: w574 -> [_ w633]
            frame False {
            }
            frame True {
              n513 = Insert Into Array(array=w635, new element=w633) -> (w634:dbl[][])  [unwired: 2 in]
            }
          }
          n514 = while {
            tunnel: w600 -> [w729]
            tunnel: w604 -> [w746]
            tunnel: w603 -> [w745]
            tunnel: [w736] -> w602
            tunnel: w582 -> [w735]
            tunnel: w582 -> [w730]
            tunnel: w573 -> [w728]
            i -> [w780]
            stop <- w725 stop-if-true
            n515 = for {
              tunnel: w746 -> [w1040] mode=indexing
              shift-right: [w1037] -> w731
              shift-left: TRUE -> [w1041]
              n516 = Equal?(x=w1040, y="") -> (x = y?=w1038:bool)
              n517 = case shown="True" w1038 {
                tunnel: w1041 -> [_ w1043]
                tunnel: [FALSE w1043] -> w1037
                frame False {
                }
                frame True {
                }
              }
            }
            n518 = Wait (ms)(milliseconds to wait=u32 100 ("Zu wartende ms")) -> ()  [unwired: 1 out]
            n519 = Multiply(x="Zoom from end", y=-1.0) -> (x*y=w764:dbl)
            n520 = Add(x="Zoom from start", y=w764) -> (x+y=w775:dbl)
            n521 = feedback #4() -> (w770:dbl)  [unwired: 1 in]
            n522 = Greater Or Equal?(x=w775, y=0.0) -> (x >= y?=w773:bool)
            n523 = Less?(x=w735, y=2) -> (x < y?=w733:bool)
            n524 = case shown="True" w773 {
              tunnel: "Zoom from start" -> [w1052 w1055]
              tunnel: [w1051 w1055] -> w771
              tunnel: w770 -> [w1051 w1057]
              tunnel: "Zoom from end" -> [_ w1054]
              tunnel: [w1052 w1055] -> w763
              tunnel: [w1050 w1053] -> w762
              tunnel: "Zoom from end" -> [w1050 w1053]
              frame False {
              }
              frame True {
                n525 = Not Equal?(x=w1057, y=w1055) -> (x != y?=w1056:bool)
                n526 = case shown="False" w1056 {
                  tunnel: w1055 -> [_ w1059]
                  tunnel: w1054 -> [w1058 _]
                  frame False {
                    n527 = local write "Zoom from start"(w1058) -> ()
                  }
                  frame True {
                    n528 = local write "Zoom from end"(w1059) -> ()
                  }
                }
              }
            }
            n529 = feedback-in #4(w771) -> ()
            n530 = Or(x=w731, y=w733) -> (x .or. y?=w732:bool)
            n531 = case shown="False" w732 {
              tunnel: w745 -> [w1033 w1036]
              tunnel: [w1035 w1036] -> w736
              tunnel: w746 -> [w1034 _]
              frame False {
                n532 = Insert Into Array(array=w1033, new element=w1034) -> (w1035:string[])  [unwired: 1 in]
              }
              frame True {
              }
            }
            n533 = Array Size(array=w736) -> (size(s)=w742:i32)
            n534 = Array Subset(array=w736, index=1 ("Index")) -> (w750:string[])  [unwired: 1 in]
            n535 = Subtract(x=w762, y=w763) -> (x-y=w769:dbl)
            n536 = Divide(x=w742, y=10) -> (x/y=w740:dbl)
            n537 = for {
              tunnel: w750 -> [w1046] mode=indexing
              shift-right: [w1049] -> w748
              shift-left: dbl[] [] -> [w1048]
              n538 = Match Pattern(string=w1046, regular expression="\t") -> (before substring=w1044:string)  [unwired: 1 in, 3 out]
              n539 = Fract/Exp String To Number(string=w1044) -> (number=w1047:dbl)  [unwired: 3 in, 1 out]
              n540 = Insert Into Array(array=w1048, new element=w1047) -> (w1049:dbl[])  [unwired: 1 in]
            }
            n541 = Index Array(array=w729, index (col)=0 ("Deaktivierter Index (Spalte)")) -> (element=w777:dbl[])  [unwired: 1 in]
            n542 = Multiply(x=w740, y="Bildlaufleiste") -> (x*y=w738:dbl)
            n543 = Divide(x=w763, y=100.0) -> (x/y=w765:dbl)
            n544 = Divide(x=w769, y=100.0) -> (x/y=w766:dbl)
            n545 = Array Size(array=w777) -> (size(s)=w759:i32)
            n546 = Array Subset(array=w736, index=w738) -> (w737:string[])  [unwired: 1 in]
            n547 = Multiply(x=w759, y=w765) -> (x*y=w755:dbl)
            n548 = Multiply(x=w759, y=w766) -> (x*y=w758:dbl)
            n549 = Index Array(array=w728, index="TC 3") -> (element=w727:bool)
            n550 = Add(x=w758, y=2.0) -> (x+y=w756:dbl)
            n551 = Subtract(x=w755, y=2.0) -> (x-y=w753:dbl)
            n552 = for {
              shift-right: [w1031] -> w743
              shift-left: "" -> [w1032]
              tunnel: w737 -> [w1029] mode=indexing
              n553 = Concatenate Strings(w1032, w1029, "\r") -> (w1031:string)
            }
            "?" <- w743
            n554 = Array Subset(array=w729, index (row)=w753, length (row)=w756) -> (w749:dbl[][])  [unwired: 2 in]
            n555 = case shown="\"SISE channel #1\", Default" "TC 3" {
              tunnel: w749 -> [w792 w872 w984 w995]
              tunnel: w748 -> [w790 w871 w952 w998]
              tunnel: w730 -> [w789 w868 w949 w990]
              tunnel: w727 -> [w786 w867 w948 w989]
              frame "SISE channel #1", Default {
                n556 = Greater Or Equal?(x=w789, y=2) -> (x >= y?=w787:bool)
                n557 = And(x=w787, y=w786) -> (x .and. y?=w785:bool)
                n558 = Index Array(array=w792, index (col)=0 ("disabled index (col)")) -> (element=w795:dbl[])  [unwired: 1 in]
                n559 = Index Array(array=w792, index (col)=1 ("disabled index (col)")) -> (element=w794:dbl[])  [unwired: 1 in]
                n560 = Index Array(array=w792, index (col)=3 ("disabled index (col)")) -> (element=w791:dbl[])  [unwired: 1 in]
                n561 = stacked-sequence {
                  tunnel: w795 -> [w799 w838]
                  tunnel: w794 -> [w818 _]
                  tunnel: w790 -> [w800 w837]
                  tunnel: w791 -> [_ w836]
                  tunnel: w785 -> [w798 w832]
                  frame #0 {
                    n562 = Array Max & Min(array=w799) -> (max value=w810:dbl, min value=w809:dbl)  [unwired: 2 out]
                    n563 = Divide(x="Range limit\nS1.1 (mV)", y=2.0) -> (x/y=w828:dbl)
                    n564 = Divide(x="Range limit\nS1.1 (mV)", y=2.05) -> (x/y=w829:dbl)
                    n565 = Add(x="Base line\nS1.1 (mV)", y=w828) -> (x+y=w801:dbl)
                    n566 = Subtract(x="Base line\nS1.1 (mV)", y=w828) -> (x-y=w802:dbl)
                    n567 = Subtract(x="Base line\nS1.1 (mV)", y=w829) -> (x-y=w808:dbl)
                    n568 = call "EventstoGraph (SubVI).vi"("Numerisch 2"=w809, "Array 3"=w800, "Numerisch"=w810, "Array (Eingang)"=dbl[][] [], "Numerisch 3"=w808) -> ("Array (Ausgang)"=w812:dbl[][])  [unwired: 6 in]
                    n569 = Array Max & Min(array=w799) -> (max value=w824:dbl, min value=w825:dbl)  [unwired: 2 out]
                    n570 = call "GraphLimit01.vi"("Numeric 2"=w802, "Numeric"=w801, "Array in"=w818, "Array 3"=dbl[] []) -> ("Array out"=w817:dbl[])  [unwired: 7 in]
                    n571 = Build Array("Base line\nS1.1 (mV)", "Base line\nS1.1 (mV)") -> (w821:dbl[])
                    n572 = Build Array(w824, w825) -> (w822:dbl[])
                    n573 = Build Array(w801, w802) -> (w823:dbl[])
                    n574 = Index Array(array=w812, index (col)=0 ("Index (Zeile)")) -> (element=w813:dbl[])  [unwired: 1 in]
                    n575 = Index Array(array=w812, index (col)=1 ("Index (Zeile)")) -> (element=w811:dbl[])  [unwired: 1 in]
                    n576 = Bundle(w822, w823) -> (w805:cluster{dbl[], dbl[]})  [unwired: 1 in]
                    n577 = Bundle(w822, w821) -> (w806:cluster{dbl[], dbl[]})  [unwired: 1 in]
                    n578 = Bundle(w799, "Array out"=w817) -> (w804:cluster{dbl[], "Array out":dbl[]})  [unwired: 1 in]
                    n579 = Bundle("Array (Ausgang)"=w813, "Array (Ausgang)"=w811) -> (w803:T9)  [unwired: 1 in]
                    n580 = Build Array(w806, w805, w804, w803) -> (w807:T10)
                    n581 = case shown="True" w798 {
                      tunnel: w807 -> [_ w831]
                      frame False {
                      }
                      frame True {
                        "V-SISE channel 1" <- w831
                      }
                    }
                  }
                  frame #1 {
                    n582 = Array Max & Min(array=w838) -> (max value=w847:dbl, min value=w846:dbl)  [unwired: 2 out]
                    n583 = Divide(x="Range limit\nS1.2 mV", y=2.0) -> (x/y=w863:dbl)
                    n584 = Divide(x="Range limit\nS1.2 mV", y=2.05) -> (x/y=w864:dbl)
                    n585 = Add(x="Base line \nS1.2 (mV)", y=w863) -> (x+y=w839:dbl)
                    n586 = Subtract(x="Base line \nS1.2 (mV)", y=w863) -> (x-y=w840:dbl)
                    n587 = Subtract(x="Base line \nS1.2 (mV)", y=w864) -> (x-y=w845:dbl)
                    n588 = call "EventstoGraph (SubVI).vi"("Numerisch 2"=w846, "Array 3"=w837, "Numerisch"=w847, "Array (Eingang)"=dbl[][] [], "Numerisch 3"=w845) -> ("Array (Ausgang)"=w849:dbl[][])  [unwired: 6 in]
                    n589 = Array Max & Min(array=w838) -> (max value=w859:dbl, min value=w860:dbl)  [unwired: 2 out]
                    n590 = call "GraphLimit01.vi"("Numeric 2"=w840, "Numeric"=w839, "Array in"=w836, "Array 3"=dbl[] []) -> ("Array out"=w854:dbl[])  [unwired: 7 in]
                    n591 = Build Array("Base line \nS1.2 (mV)", "Base line \nS1.2 (mV)") -> (w856:dbl[])
                    n592 = Build Array(w859, w860) -> (w857:dbl[])
                    n593 = Build Array(w839, w840) -> (w858:dbl[])
                    n594 = Index Array(array=w849, index (col)=0 ("Index (Zeile)")) -> (element=w850:dbl[])  [unwired: 1 in]
                    n595 = Index Array(array=w849, index (col)=1 ("Index (Zeile)")) -> (element=w848:dbl[])  [unwired: 1 in]
                    n596 = Bundle(w857, w858) -> (w843:cluster{dbl[], dbl[]})  [unwired: 1 in]
                    n597 = Bundle(w857, w856) -> (w844:cluster{dbl[], dbl[]})  [unwired: 1 in]
                    n598 = Bundle(w838, "Array out"=w854) -> (w842:cluster{dbl[], "Array out":dbl[]})  [unwired: 1 in]
                    n599 = Bundle("Array (Ausgang)"=w850, "Array (Ausgang)"=w848) -> (w841:T9)  [unwired: 1 in]
                    n600 = Build Array(w844, w843, w842, w841) -> (w833:T10)
                    n601 = case shown="True" w832 {
                      tunnel: w833 -> [_ w865]
                      frame False {
                      }
                      frame True {
                        "dV-SISE channel 1" <- w865
                      }
                    }
                  }
                }
              }
              frame "SISE channel #2" {
                n602 = Greater Or Equal?(x=w868, y=2) -> (x >= y?=w870:bool)
                n603 = And(x=w870, y=w867) -> (x .and. y?=w866:bool)
                n604 = Index Array(array=w872, index (col)=0 ("disabled index (col)")) -> (element=w876:dbl[])  [unwired: 1 in]
                n605 = Index Array(array=w872, index (col)=2 ("disabled index (col)")) -> (element=w877:dbl[])  [unwired: 1 in]
                n606 = Index Array(array=w872, index (col)=4 ("disabled index (col)")) -> (element=w878:dbl[])  [unwired: 1 in]
                n607 = stacked-sequence {
                  tunnel: w876 -> [w880 w919]
                  tunnel: w877 -> [w899 _]
                  tunnel: w871 -> [w881 w918]
                  tunnel: w878 -> [_ w917]
                  tunnel: w866 -> [w879 w913]
                  frame #0 {
                    n608 = Array Max & Min(array=w880) -> (max value=w891:dbl, min value=w890:dbl)  [unwired: 2 out]
                    n609 = Divide(x="Range limit\nS2.1 (mV)", y=2.0) -> (x/y=w909:dbl)
                    n610 = Divide(x="Range limit\nS2.1 (mV)", y=2.05) -> (x/y=w910:dbl)
                    n611 = Add(x="Base line\nS2.1 (mV)", y=w909) -> (x+y=w882:dbl)
                    n612 = Subtract(x="Base line\nS2.1 (mV)", y=w909) -> (x-y=w883:dbl)
                    n613 = Subtract(x="Base line\nS2.1 (mV)", y=w910) -> (x-y=w889:dbl)
                    n614 = call "EventstoGraph (SubVI).vi"("Numerisch 2"=w890, "Array 3"=w881, "Numerisch"=w891, "Array (Eingang)"=dbl[][] [], "Numerisch 3"=w889) -> ("Array (Ausgang)"=w893:dbl[][])  [unwired: 6 in]
                    n615 = Array Max & Min(array=w880) -> (max value=w905:dbl, min value=w906:dbl)  [unwired: 2 out]
                    n616 = call "GraphLimit01.vi"("Numeric 2"=w883, "Numeric"=w882, "Array in"=w899, "Array 3"=dbl[] []) -> ("Array out"=w898:dbl[])  [unwired: 7 in]
                    n617 = Build Array("Base line\nS2.1 (mV)", "Base line\nS2.1 (mV)") -> (w902:dbl[])
                    n618 = Build Array(w905, w906) -> (w903:dbl[])
                    n619 = Build Array(w882, w883) -> (w904:dbl[])
                    n620 = Index Array(array=w893, index (col)=0 ("Index (Zeile)")) -> (element=w894:dbl[])  [unwired: 1 in]
                    n621 = Index Array(array=w893, index (col)=1 ("Index (Zeile)")) -> (element=w892:dbl[])  [unwired: 1 in]
                    n622 = Bundle(w903, w904) -> (w886:cluster{dbl[], dbl[]})  [unwired: 1 in]
                    n623 = Bundle(w903, w902) -> (w887:cluster{dbl[], dbl[]})  [unwired: 1 in]
                    n624 = Bundle(w880, "Array out"=w898) -> (w885:cluster{dbl[], "Array out":dbl[]})  [unwired: 1 in]
                    n625 = Bundle("Array (Ausgang)"=w894, "Array (Ausgang)"=w892) -> (w884:T9)  [unwired: 1 in]
                    n626 = Build Array(w887, w886, w885, w884) -> (w888:T10)
                    n627 = case shown="True" w879 {
                      tunnel: w888 -> [_ w912]
                      frame False {
                      }
                      frame True {
                        "V-SISE channel 2" <- w912
                      }
                    }
                  }
                  frame #1 {
                    n628 = Array Max & Min(array=w919) -> (max value=w928:dbl, min value=w927:dbl)  [unwired: 2 out]
                    n629 = Divide(x="Range limit\nS2.2 (mV)", y=2.0) -> (x/y=w944:dbl)
                    n630 = Divide(x="Range limit\nS2.2 (mV)", y=2.05) -> (x/y=w945:dbl)
                    n631 = Add(x="Base line \nS2.2 (mV)", y=w944) -> (x+y=w920:dbl)
                    n632 = Subtract(x="Base line \nS2.2 (mV)", y=w944) -> (x-y=w921:dbl)
                    n633 = Subtract(x="Base line \nS2.2 (mV)", y=w945) -> (x-y=w926:dbl)
                    n634 = call "EventstoGraph (SubVI).vi"("Numerisch 2"=w927, "Array 3"=w918, "Numerisch"=w928, "Array (Eingang)"=dbl[][] [], "Numerisch 3"=w926) -> ("Array (Ausgang)"=w930:dbl[][])  [unwired: 6 in]
                    n635 = Array Max & Min(array=w919) -> (max value=w940:dbl, min value=w941:dbl)  [unwired: 2 out]
                    n636 = call "GraphLimit01.vi"("Numeric 2"=w921, "Numeric"=w920, "Array in"=w917, "Array 3"=dbl[] []) -> ("Array out"=w935:dbl[])  [unwired: 7 in]
                    n637 = Build Array("Base line \nS2.2 (mV)", "Base line \nS2.2 (mV)") -> (w937:dbl[])
                    n638 = Build Array(w940, w941) -> (w938:dbl[])
                    n639 = Build Array(w920, w921) -> (w939:dbl[])
                    n640 = Index Array(array=w930, index (col)=0 ("Index (Zeile)")) -> (element=w931:dbl[])  [unwired: 1 in]
                    n641 = Index Array(array=w930, index (col)=1 ("Index (Zeile)")) -> (element=w929:dbl[])  [unwired: 1 in]
                    n642 = Bundle(w938, w939) -> (w924:cluster{dbl[], dbl[]})  [unwired: 1 in]
                    n643 = Bundle(w938, w937) -> (w925:cluster{dbl[], dbl[]})  [unwired: 1 in]
                    n644 = Bundle(w919, "Array out"=w935) -> (w923:cluster{dbl[], "Array out":dbl[]})  [unwired: 1 in]
                    n645 = Bundle("Array (Ausgang)"=w931, "Array (Ausgang)"=w929) -> (w922:T9)  [unwired: 1 in]
                    n646 = Build Array(w925, w924, w923, w922) -> (w914:T10)
                    n647 = case shown="True" w913 {
                      tunnel: w914 -> [_ w946]
                      frame False {
                      }
                      frame True {
                        "dV-SISE channel 2" <- w946
                      }
                    }
                  }
                }
              }
              frame "V channel #1" {
                n648 = Greater Or Equal?(x=w949, y=2) -> (x >= y?=w951:bool)
                n649 = And(x=w951, y=w948) -> (x .and. y?=w947:bool)
                n650 = Index Array(array=w984, index (col)=0 ("disabled index (col)")) -> (element=w953:dbl[])  [unwired: 1 in]
                n651 = Index Array(array=w984, index (col)=5 ("disabled index (col)")) -> (element=w954:dbl[])  [unwired: 1 in]
                n652 = Array Max & Min(array=w953) -> (max value=w964:dbl, min value=w963:dbl)  [unwired: 2 out]
                n653 = Divide(x="Range limit\nV1 (V)", y=2.0) -> (x/y=w981:dbl)
                n654 = Divide(x="Range limit\nV1 (V)", y=2.05) -> (x/y=w982:dbl)
                n655 = Add(x="Base line\nV1 (V)", y=w981) -> (x+y=w955:dbl)
                n656 = Subtract(x="Base line\nV1 (V)", y=w981) -> (x-y=w956:dbl)
                n657 = Subtract(x="Base line\nV1 (V)", y=w982) -> (x-y=w962:dbl)
                n658 = call "EventstoGraph (SubVI).vi"("Numerisch 2"=w963, "Array 3"=w952, "Numerisch"=w964, "Array (Eingang)"=dbl[][] [], "Numerisch 3"=w962) -> ("Array (Ausgang)"=w966:dbl[][])  [unwired: 6 in]
                n659 = Array Max & Min(array=w953) -> (max value=w977:dbl, min value=w978:dbl)  [unwired: 2 out]
                n660 = call "GraphLimit01.vi"("Numeric 2"=w956, "Numeric"=w955, "Array in"=w954, "Array 3"=dbl[] []) -> ("Array out"=w971:dbl[])  [unwired: 7 in]
                n661 = Build Array("Base line\nV1 (V)", "Base line\nV1 (V)") -> (w974:dbl[])
                n662 = Build Array(w977, w978) -> (w975:dbl[])
                n663 = Build Array(w955, w956) -> (w976:dbl[])
                n664 = Index Array(array=w966, index (col)=0 ("Index (Zeile)")) -> (element=w967:dbl[])  [unwired: 1 in]
                n665 = Index Array(array=w966, index (col)=1 ("Index (Zeile)")) -> (element=w965:dbl[])  [unwired: 1 in]
                n666 = Bundle(w975, w976) -> (w959:cluster{dbl[], dbl[]})  [unwired: 1 in]
                n667 = Bundle(w975, w974) -> (w960:cluster{dbl[], dbl[]})  [unwired: 1 in]
                n668 = Bundle(w953, "Array out"=w971) -> (w958:cluster{dbl[], "Array out":dbl[]})  [unwired: 1 in]
                n669 = Bundle("Array (Ausgang)"=w967, "Array (Ausgang)"=w965) -> (w957:T9)  [unwired: 1 in]
                n670 = Build Array(w960, w959, w958, w957) -> (w961:T10)
                n671 = case shown="True" w947 {
                  tunnel: w961 -> [_ w987]
                  frame False {
                  }
                  frame True {
                    "Voltage channel 1" <- w987
                  }
                }
              }
              frame "V channel #2" {
                n672 = Greater Or Equal?(x=w990, y=2) -> (x >= y?=w991:bool)
                n673 = And(x=w991, y=w989) -> (x .and. y?=w988:bool)
                n674 = Index Array(array=w995, index (col)=0 ("disabled index (col)")) -> (element=w993:dbl[])  [unwired: 1 in]
                n675 = Index Array(array=w995, index (col)=6 ("disabled index (col)")) -> (element=w994:dbl[])  [unwired: 1 in]
                n676 = Array Max & Min(array=w993) -> (max value=w1008:dbl, min value=w1007:dbl)  [unwired: 2 out]
                n677 = Divide(x="Range limit\nV2 (V)", y=2.0) -> (x/y=w1025:dbl)
                n678 = Divide(x="Range limit\nV2 (V)", y=2.05) -> (x/y=w1026:dbl)
                n679 = Add(x="Base line\nV2 (V)", y=w1025) -> (x+y=w999:dbl)
                n680 = Subtract(x="Base line\nV2 (V)", y=w1025) -> (x-y=w1000:dbl)
                n681 = Subtract(x="Base line\nV2 (V)", y=w1026) -> (x-y=w1006:dbl)
                n682 = call "EventstoGraph (SubVI).vi"("Numerisch 2"=w1007, "Array 3"=w998, "Numerisch"=w1008, "Array (Eingang)"=dbl[][] [], "Numerisch 3"=w1006) -> ("Array (Ausgang)"=w1010:dbl[][])  [unwired: 6 in]
                n683 = Array Max & Min(array=w993) -> (max value=w1021:dbl, min value=w1022:dbl)  [unwired: 2 out]
                n684 = call "GraphLimit01.vi"("Numeric 2"=w1000, "Numeric"=w999, "Array in"=w994, "Array 3"=dbl[] []) -> ("Array out"=w1015:dbl[])  [unwired: 7 in]
                n685 = Build Array("Base line\nV2 (V)", "Base line\nV2 (V)") -> (w1018:dbl[])
                n686 = Build Array(w1021, w1022) -> (w1019:dbl[])
                n687 = Build Array(w999, w1000) -> (w1020:dbl[])
                n688 = Index Array(array=w1010, index (col)=0 ("Index (Zeile)")) -> (element=w1011:dbl[])  [unwired: 1 in]
                n689 = Index Array(array=w1010, index (col)=1 ("Index (Zeile)")) -> (element=w1009:dbl[])  [unwired: 1 in]
                n690 = Bundle(w1019, w1020) -> (w1003:cluster{dbl[], dbl[]})  [unwired: 1 in]
                n691 = Bundle(w1019, w1018) -> (w1004:cluster{dbl[], dbl[]})  [unwired: 1 in]
                n692 = Bundle(w993, "Array out"=w1015) -> (w1002:cluster{dbl[], "Array out":dbl[]})  [unwired: 1 in]
                n693 = Bundle("Array (Ausgang)"=w1011, "Array (Ausgang)"=w1009) -> (w1001:T9)  [unwired: 1 in]
                n694 = Build Array(w1004, w1003, w1002, w1001) -> (w1005:T10)
                n695 = case shown="True" w988 {
                  tunnel: w1005 -> [_ w1028]
                  frame False {
                  }
                  frame True {
                    "Voltage channel 2" <- w1028
                  }
                }
              }
            }
            n696 = local read "Record period (round at 5s)"() -> (w779:dbl)
            n697 = local read "Stop recording 2"() -> (w723:bool)
            n698 = Multiply(x=w779, y=10.0) -> (x*y=w783:dbl)
            n699 = Subtract(x=w783, y=10.0) -> (x-y=w781:dbl)
            n700 = Greater Or Equal?(x=w780, y=w781) -> (x >= y?=w724:bool)
            n701 = Or(x=w723, y=w724) -> (x .or. y?=w725:bool)
          }
        }
        n702 = disable-structure shown="Disabled" {
          disable-tunnel: w522 -> [w569 _]
          disable-tunnel: w521 -> [w568 _]
          frame Disabled {
            n703 = call <vilib>:"DAQmx Stop Task.vi"("task/channels in"=w569, "error in"=w568) -> ()  [unwired: 12 in, 2 out]
          }
          frame Enabled {
          }
        }
        n704 = Unbundle(w521) -> ("status"=w558:bool, "code"=w557:i32, "source"=w556:string)
        n705 = Close File(refnum=w519, error in=w520) -> ()  [unwired: 2 out]
        n706 = Unbundle(w520) -> ("status"=w538:bool, "code"=w537:i32, "source"=w536:string)
        n707 = Bundle("task out"=w522, "status"=w558, "code"=w557, "source"=w556) -> (w555:T5)  [unwired: 1 in]
        n708 = Bundle("refnum out"=w519, "status"=w538, "code"=w537, "source"=w536) -> (w535:T4)  [unwired: 1 in]
        n709 = Release Queue(queue=w553, error in (no error)=w552) -> ()  [unwired: 1 in, 3 out]
      }
      frame 2 {
        n710 = while {
          tunnel: w1648 -> [w1656]
          tunnel: [w1655] -> w1647
          stop <- w1659 stop-if-true
          n711 = Wait (ms)(milliseconds to wait=u32 100 ("Zu wartende ms")) -> ()  [unwired: 1 out]
          n712 = case shown="True" "Stop programm" {
            tunnel: w1656 -> [w1661 _]
            tunnel: [w1661 TRUE] -> w1655
            frame False {
            }
            frame True {
            }
          }
          n713 = Or(x="New measurement", y="Stop programm") -> (x .or. y?=w1659:bool)
        }
      }
    }
    "Registerkarte" <- w27
  }
